vi "NI_cDAQ.vi"(7 "simulazione":bool, 8 "error in (no error)":errorcluster, 10 "banco":i32, 11 "Queue Name":string="NIcDAQ_Q") -> (0 "error out":errorcluster, 2 "Stopped":bool)   [LabVIEW 2019]
uses:
  TypeDef/Cluster NI.ctl
  cDAQ_PLC Folder/controls/StatoAO_cdaq.ctl
  cDAQ_PLC Folder/controls/statoDO_Cdaq.ctl
  cDAQ_PLC Folder/IN_Cluster.ctl
  cDAQ_PLC Folder/OUT_CLUSTER.ctl
  <vilib>/addons/_NISVFA/_Shared subVIs/Controls/svc_Channel Info.ctl
  <vilib>/addons/_NISVFA/_Shared subVIs/Controls/svc_Engineering Units Text Ring.ctl
  <vilib>/addons/_NISVFA/_Shared subVIs/Controls/svc_Weighting Filter Text Ring.ctl
  <vilib>/addons/_NISVFA/_Shared subVIs/Controls/svc_Window.ctl
  TypeDef/DEVICE NAME.ctl
  TypeDef/CLUSTER AI SIM.ctl
  <vilib>/DAQmx/read.llb/DAQmx Read (Counter DBL 1Chan 1Samp).vi
  <vilib>/DAQmx/read.llb/DAQmx Read (Analog 1D Wfm NChan NSamp).vi
  <vilib>/Analysis/baseanly.llb/Mean (DBL).vi
  <vilib>/DAQmx/write.llb/DAQmx Write (Digital 1D Bool NChan 1Samp 1Line).vi
  <vilib>/DAQmx/write.llb/DAQmx Write (Analog 1D DBL NChan 1Samp).vi
  <vilib>/Utility/file.llb/Read From Spreadsheet File (string).vi
  <vilib>/Utility/file.llb/Write To Spreadsheet File (string).vi
  <vilib>/DAQmx/miscellaneous.llb/DAQmx Fill In Error Info.vi
  Globals.vi
  <vilib>/Utility/file.llb/Read From Spreadsheet File (DBL).vi
  <vilib>/Analysis/NI_AALBase.lvlib
  cDAQ_PLC Folder/SubVI/EXIT.vi
  Global allarme combinazione DO.vi
  <vilib>/addons/Sound and Vibration/svt_Calibration/SoundVib_Calibration.lvlib
  <vilib>/measure/NI_MAPro.lvlib
  <vilib>/measure/NI_MABase.lvlib
  rpm nominali global.vi
  <resource>/objmgr/daqmx.rc
  <vilib>/DAQmx/read.llb/DAQmx Read (Analog 1D DBL NChan 1Samp).vi
  <vilib>/DAQmx/read.llb/DAQmx Read (Analog Wfm 1Chan NSamp).vi
  <vilib>/DAQmx/configure/timing.llb/DAQmx Timing (Sample Clock).vi
  <vilib>/addons/Sound and Vibration/svt_Calibration/SVL Scale Voltage to EU (1 Ch).vi
  <vilib>/addons/_NISVFA/_Spectrum Processing/SVFA Spectrum Peak Search (1 Ch).vi
  <vilib>/addons/_NISVFA/_Subset FFT/SVFA Power Spectrum Subset (1 Ch).vi
panel:
  in  "element":dbl[](array[numeric])
  in  "SET AO":bool
  out "EXIT 2":bool=TRUE
  out "error AO 2":errorcluster
  out "# pending insert 4":i32
  out "t ciclo effettivo AO 2":u32
  out "AO cdaq [0-10V]":T1
  out "x-y 2":u32
  out "Array":dbl[](array[numeric])
  out "error DO 2":errorcluster
  out "statoDO 2":T2
  out "# pending insert 3":i32
  out "Numeric 2":i32
  out "stop":bool
  in  "dB On (T)":bool=TRUE
  out "Letture":T3 {"Stato uscite"."AO" format="%f%0.2f"; "AI2" format="%#_6f"; "TC" format="%#_4f"; "AI1" format="%#_6f"}
  out "AO cdaq 4-20mA":T1
  out "Temperature [°C]":T5
  out "Contatori [rpm]":cluster{"RPM 1":dbl, "RPM 2":dbl}
  out "error AO":errorcluster
  out "x-y":u32
  out "# pending insert 2":i32
  out "t ciclo effettivo AO":u32
  out "SampleRate":dbl
  out "subarray":string[](array[string])
  out "all rows":string[][](array[string])
  out "N°samples":i32
  out "appended path":path
  out "SampleMode":i32
  in  "Tab Control":T6(tab)
  in  "ESEGUI SOLO IL VI":bool
  out "LOOP TIME (ms)":u32
  out "Cluster READ":T7 {"AI (4-20mA)"."AI 15" format="%#_6f"; "AI (4-20mA)"."AI 14" format="%#_6f"; "AI (4-20mA)"."AI 13" format="%#_6f"; "AI (4-20mA)"."AI 11" format="%#_6f"; "AI (4-20mA)"."AI 10" format="%#_6f"; "AI (4-20mA)"."AI 9" format="%#_6f"; "AI (4-20mA)"."AI 4" format="%#_6f"; "AI (4-20mA)"."AI 12" format="%#_6f"; "AI (4-20mA)"."AI 0" format="%#_6f"; "AI (4-20mA)"."AI 1" format="%#_6f"; "AI (4-20mA)"."AI 2" format="%#_6f"; "AI (4-20mA)"."AI 3" format="%#_6f"; "AI (4-20mA)"."AI 5" format="%#_6f"; "AI (4-20mA)"."AI 6" format="%#_6f"; "AI (4-20mA)"."AI 7" format="%#_6f"; "AI (4-20mA)"."AI 8" format="%#_6f"; "AI (0-10V)"."AI 31" format="%#_6f"; "AI (0-10V)"."AI 30" format="%#_6f"; "AI (0-10V)"."AI 29" format="%#_6f"; "AI (0-10V)"."AI 28" format="%#_6f"; "AI (0-10V)"."AI 27" format="%#_6f"; "AI (0-10V)"."AI 26" format="%#_6f"; "AI (0-10V)"."AI 25" format="%#_6f"; "AI (0-10V)"."AI 24" format="%#_6f"; "AI (0-10V)"."AI 23" format="%#_6f"; "AI (0-10V)"."AI 22" format="%#_6f"; "AI (0-10V)"."AI 21" format="%#_6f"; "AI (0-10V)"."AI 20" format="%#_6f"; "AI (0-10V)"."AI 19" format="%#_6f"; "AI (0-10V)"."AI 18" format="%#_6f"; "AI (0-10V)"."AI 17" format="%#_6f"; "AI (0-10V)"."AI 16" format="%#_6f"; "AI (0-10V)"."AI 15" format="%#.3f"; "AI (0-10V)"."AI 14" format="%#.3f"; "AI (0-10V)"."AI 13" format="%#.3f"; "AI (0-10V)"."AI 11" format="%#.3f"; "AI (0-10V)"."AI 10" format="%#.3f"; "AI (0-10V)"."AI 9" format="%#.3f"; "AI (0-10V)"."AI 4" format="%#.3f"; "AI (0-10V)"."AI 12" format="%#.3f"; "AI (0-10V)"."AI 0" format="%#.3f"; "AI (0-10V)"."AI 1" format="%#.3f"; "AI (0-10V)"."AI 2" format="%#.3f"; "AI (0-10V)"."AI 3" format="%#.3f"; "AI (0-10V)"."AI 5" format="%#.3f"; "AI (0-10V)"."AI 6" format="%#.3f"; "AI (0-10V)"."AI 7" format="%#.3f"; "AI (0-10V)"."AI 8" format="%#.3f"}
  out "frequency":dbl
  out "error TC":errorcluster
  out "STATO":string
  out "variant":variant
  out "Array nomi moduli":string[](array[string])
  out "Cluster TASK":T9
  in  "lower limit":dbl=1.0 format="%#_13g"
  in  "upper limit":dbl=10000.0 format="%#_13g"
  in  "campioni media rpm":i32=3
  in  "timeout":dbl=0.5 format="%#_13g"
  out "Frequenza":dbl
  out "error in (no error) 2":errorcluster
  out "error out 3":errorcluster
  out "CTR error 2":errorcluster
  out "NI9203":errorcluster caption="error out"
  out "NI9265":errorcluster
  out "CTR TASK":errorcluster caption="error out"
  out "NI9215":errorcluster caption="ni 9215"
  in  "Boolean":bool
  in  "DI.DigFltr.Enable":bool=TRUE
  in  "DI.DigFltr.MinPulseWidth":dbl=6.4e-06
  out "Numeric":i32
  in  "SALVA IMP FILTRI 0-10V":bool
  out "Not filtered 4-20mA":waveform(dbl)[](graph)
  out "Filtered 4-20mA":waveform(dbl)[](graph)
  in  "Impostazioni filtri digitali su canali 4-20mA":T10(array[cluster])=[{"filter?"=FALSE, "low cutoff freq: fl"=0.12500000000000006, "order"=2}, {"filter?"=FALSE, "low cutoff freq: fl"=0.12500000000000006, "order"=2}, {"filter?"=FALSE, "low cutoff freq: fl"=0.12500000000000006, "order"=2}, {"filter?"=FALSE, "low cutoff freq: fl"=0.12500000000000006, "order"=2}, {"filter?"=FALSE, "low cutoff freq: fl"=0.12500000000000006, "order"=2}, {"filter?"=FALSE, "low cutoff freq: fl"=0.12500000000000006, "order"=2}, {"filter?"=FALSE, "low cutoff freq: fl"=0.12500000000000006, "order"=2}, {"filter?"=FALSE, "low cutoff freq: fl"=0.12500000000000006, "order"=2}, {"filter?"=FALSE, "low cutoff freq: fl"=0.12500000000000006, "order"=2}, {"filter?"=FALSE, "low cutoff freq: fl"=0.12500000000000006, "order"=2}, {"filter?"=FALSE, "low cutoff freq: fl"=0.12500000000000006, "order"=2}, {"filter?"=FALSE, "low cutoff freq: fl"=0.12500000000000006, "order"=2}, {"filter?"=FALSE, "low cutoff freq: fl"=0.12500000000000006, "order"=2}, {"filter?"=FALSE, "low cutoff freq: fl"=0.12500000000000006, "order"=2}, {"filter?"=FALSE, "low cutoff freq: fl"=0.12500000000000006, "order"=2}, {"filter?"=FALSE, "low cutoff freq: fl"=0.12500000000000006, "order"=2}] {"low cutoff freq: fl" format="%0.4f"}
  in  "SALVA IMP FILTRI 4-20mA":bool
  in  "Impostazioni filtri digitali su canali 0-10V":T10(array[cluster])=[{"filter?"=FALSE, "low cutoff freq: fl"=0.12500000000000006, "order"=2}, {"filter?"=FALSE, "low cutoff freq: fl"=0.12500000000000006, "order"=2}, {"filter?"=FALSE, "low cutoff freq: fl"=0.12500000000000006, "order"=2}, {"filter?"=FALSE, "low cutoff freq: fl"=0.12500000000000006, "order"=2}, {"filter?"=FALSE, "low cutoff freq: fl"=0.12500000000000006, "order"=2}, {"filter?"=FALSE, "low cutoff freq: fl"=0.12500000000000006, "order"=2}, {"filter?"=FALSE, "low cutoff freq: fl"=0.12500000000000006, "order"=2}, {"filter?"=FALSE, "low cutoff freq: fl"=0.12500000000000006, "order"=2}, {"filter?"=FALSE, "low cutoff freq: fl"=0.12500000000000006, "order"=2}, {"filter?"=FALSE, "low cutoff freq: fl"=0.12500000000000006, "order"=2}, {"filter?"=FALSE, "low cutoff freq: fl"=0.12500000000000006, "order"=2}, {"filter?"=FALSE, "low cutoff freq: fl"=0.12500000000000006, "order"=2}, {"filter?"=FALSE, "low cutoff freq: fl"=0.12500000000000006, "order"=2}, {"filter?"=FALSE, "low cutoff freq: fl"=0.12500000000000006, "order"=2}, {"filter?"=FALSE, "low cutoff freq: fl"=0.12500000000000006, "order"=2}, {"filter?"=FALSE, "low cutoff freq: fl"=0.12500000000000006, "order"=2}] {"low cutoff freq: fl" format="%0.4f"}
  out "Filtered 0-10V":waveform(dbl)[](graph)
  out "Not filtered 0-10V":waveform(dbl)[](graph)
  in  "tone amplitudes":dbl[](array[numeric])=[1.0, 1.0, 1.0, 1.0] format="%.2p"
  in  "tone frequencies":dbl[](array[numeric])=[100.0, 200.0, 300.0, 400.0] format="%.2p"
  in  "averaging parameters":T11={"averaging mode"=enum."Peak hold", "weighting mode"=enum."Exponential", "number of averages"=10, "linear mode"=enum."Auto restart"}
  in  "channel info":T12={"sensor sensitivity"=100.0, "engineering units"=3, "dB reference"=2e-05, "custom label"="EU", "weighting filter"=0, "pregain"=0.0} {"pregain" format="%.2f"; "weighting filter" items=["Linear", "A-weighting", "B-weighting", "C-weighting", "ITU-R 468-4", "Dolby", "CCITT", "C-message", "Wb", "Wc", "Wd", "We", "Wf", "Wh", "Wj", "Wk", "Wm", "AES17 20 kHz lowpass", "AES17 40 kHz lowpass", "AES17 20 kHz highpass", "AES17 40 kHz highpass"]; "dB reference" format="%^.1e"; "engineering units" items=["custom..."=0, "V"=1, "A"=21, "C"=30, "pC"=31, "s"=32, "-"=29, "Pa"=2, "N"=20, "g"=3, "m/s^2"=4, "m/s"=5, "m"=6, "mm/s"=12, "mm"=13, "micron/s"=14, "micron"=15, "in/s^2"=7, "in/s"=8, "in"=9, "mil/s"=10, "mil"=11, "rad/s^2"=16, "rad/s"=17, "rad"=18, "deg/s^2"=26, "deg/s"=27, "deg"=28, "RPM"=22, "cycle/s^2"=23, "Hz"=24, "cycle"=25, "strain"=19]; "sensor sensitivity" format="%#_5f"}
  out "peaks found":i32(listbox)=-1
  out "averages completed":dbl
  out "averaging done":bool
  out "number of peaks":i32
  in  "window":T15 items=["None"=0, "Hanning"=1, "Hamming"=2, "Blackman-Harris"=3, "Exact Blackman"=4, "Blackman"=5, "Flat Top"=6, "4 Term B-Harris "=7, "7 Term B-Harris"=8, "Low Sidelobe"=9, "Force"=64, "Exponential"=65, "Blackman Nuttall"=11, "Triangle"=30, "Bartlett-Hanning"=31, "Bohman"=32, "Parzen"=33, "Welch"=34, "Kaiser"=60, "Dolph-Chebyshev"=61, "Gaussian"=62]
  out "Power Spectrum":cluster{"f0":dbl, "df":dbl, "magnitude":dbl[]}(graph)={"f0"=200.0, "df"=0.5, "magnitude"=[]}
  out "frequency range [Hz]":cluster{"start":dbl, "stop":dbl}={"start"=200.0, "stop"=2000.0} {"stop" min=0.0 format="%.2f"; "start" min=0.0 format="%.2f"}
  in  "peak search settings":T16={"single/multiple"=enum."Single Max Peak", "threshold"=inf} {"threshold" format="%.2f"}
  out "F RPM NOM":dbl
  out "Server_RPM_Nom":dbl
  in  "TOLL F-":dbl=4.0
  in  "toll F+":dbl=1.0
  out "RPM":dbl
  out "detected frequency":dbl format="%.2p"
  in  "number of samples":i32=100000
  in  "rate":dbl=40000.0 format="%0.2f"
  out "x = y?":bool
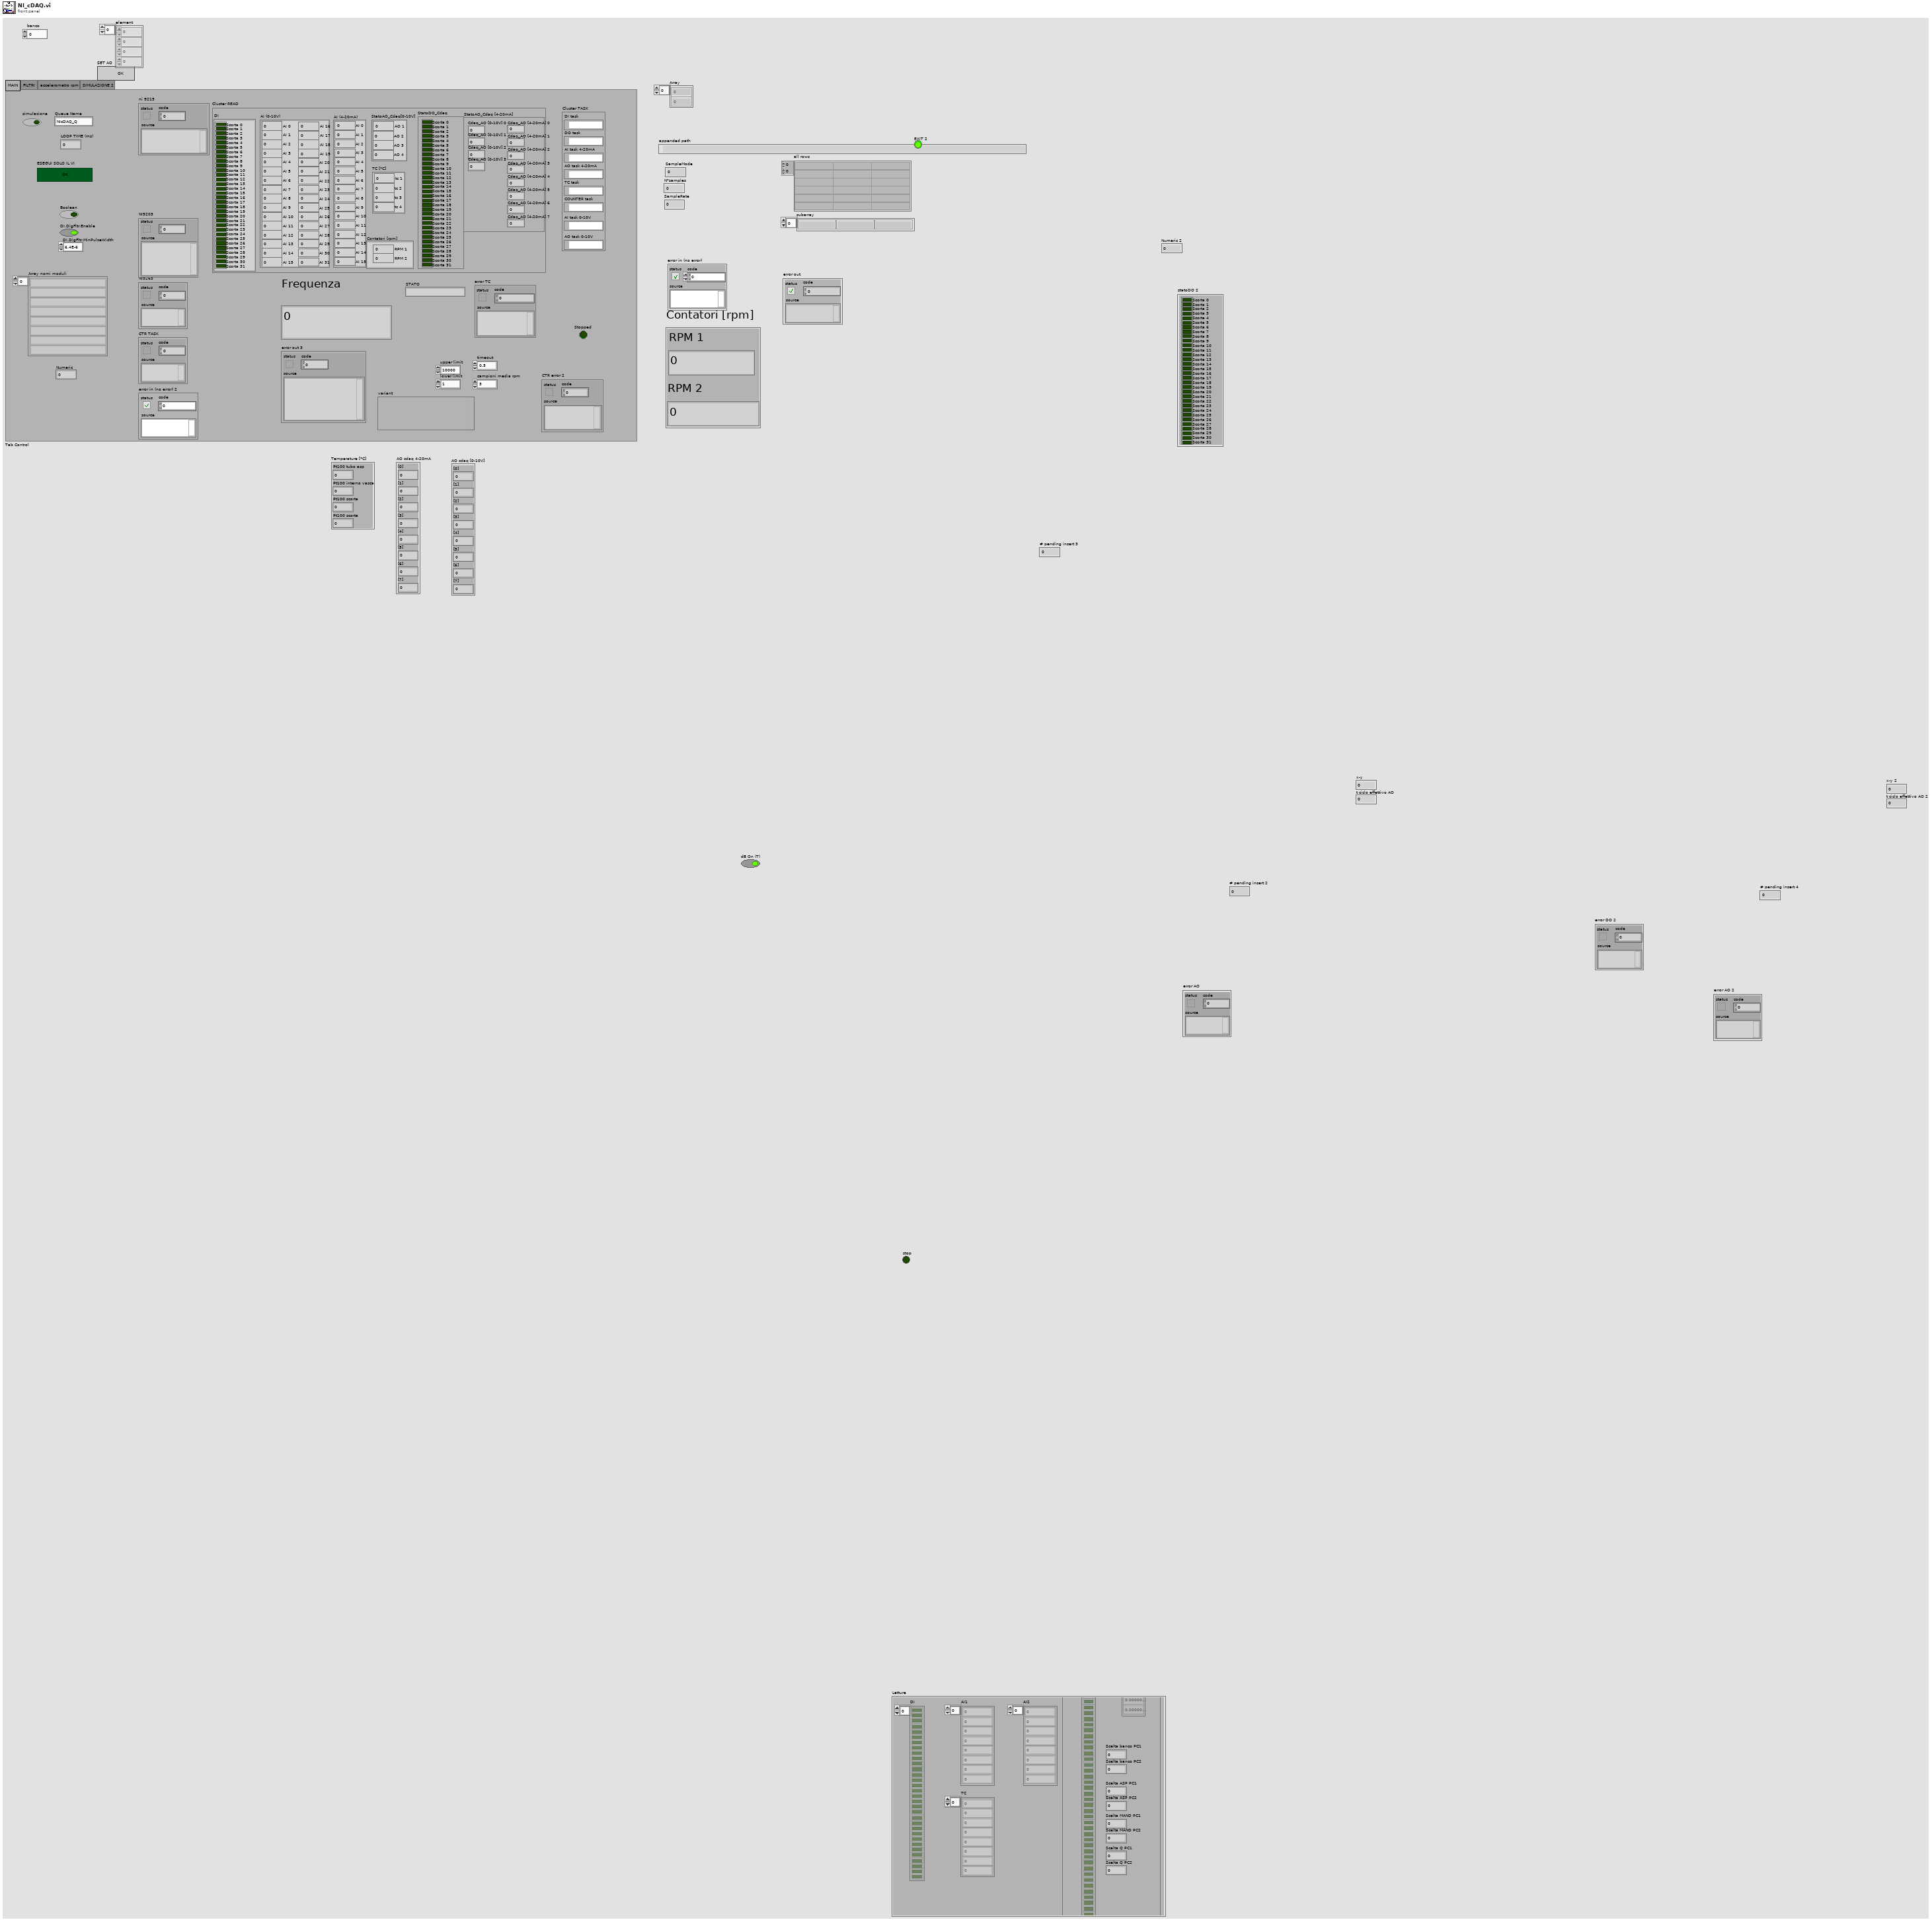
[diagram p1: front panel]
types:
  T1 = cluster{"[0]":dbl, "[1]":dbl, "[2]":dbl, "[3]":dbl, "[4]":dbl, "[5]":dbl, "[6]":dbl, "[7]":dbl}
  T2 = typedef "statoDO_Cdaq.ctl" = cluster{"Scorta 0":bool, "Scorta 1":bool, "Scorta 2":bool, "Scorta 3":bool, "Scorta 4":bool, "Scorta 5":bool, "Scorta 6":bool, "Scorta 7":bool, "Scorta 8":bool, "Scorta 9":bool, "Scorta 10":bool, "Scorta 11":bool, "Scorta 12":bool, "Scorta 13":bool, "Scorta 14":bool, "Scorta 15":bool, "Scorta 16":bool, "Scorta 17":bool, "Scorta 18":bool, "Scorta 19":bool, "Scorta 20":bool, "Scorta 21":bool, "Scorta 22":bool, "Scorta 23":bool, "Scorta 24":bool, "Scorta 25":bool, "Scorta 26":bool, "Scorta 27":bool, "Scorta 28":bool, "Scorta 29":bool, "Scorta 30":bool, "Scorta 31":bool}
  T3 = typedef "IN_Cluster.ctl" = cluster{"DI":bool[], "AI1":dbl[], "TC":dbl[], "AI2":dbl[], "Stato uscite":T4}
  T4 = typedef "OUT_CLUSTER.ctl" = cluster{"DO ":bool[], "AO":dbl[], "Scelta banco PC1":dbl, "Scelta banco PC2":dbl, "Scelta ASP PC1":dbl, "Scelta ASP PC2":dbl, "Scelta MAND PC1":dbl, "Scelta MAND PC2":dbl, "Scelta Q PC1":dbl, "Scelta Q PC2":dbl}
  T5 = cluster{"Pt100 tubo asp":dbl, "Pt100 interno vasca":dbl, "Pt100 scorta":dbl, "Pt100 scorta":dbl}
  T6 = enum32{"MAIN", "FILTRI", "accelerometro rpm", "SIMULAZIONE 2"}
  T7 = typedef "Cluster NI.ctl" = cluster{"AI (0-10V)":cluster{"AI 0":dbl, "AI 1":dbl, "AI 2":dbl, "AI 3":dbl, "AI 4":dbl, "AI 5":dbl, "AI 6":dbl, "AI 7":dbl, "AI 8":dbl, "AI 9":dbl, "AI 10":dbl, "AI 11":dbl, "AI 12":dbl, "AI 13":dbl, "AI 14":dbl, "AI 15":dbl, "AI 16":dbl, "AI 17":dbl, "AI 18":dbl, "AI 19":dbl, "AI 20":dbl, "AI 21":dbl, "AI 22":dbl, "AI 23":dbl, "AI 24":dbl, "AI 25":dbl, "AI 26":dbl, "AI 27":dbl, "AI 28":dbl, "AI 29":dbl, "AI 30":dbl, "AI 31":dbl}, "StatoAO_Cdaq[0-10V]":cluster{"AO 1":dbl, "AO 2":dbl, "AO 3":dbl, "AO 4":dbl}, "Contatori [rpm]":cluster{"RPM 1":dbl, "RPM 2":dbl}, "StatoAO_Cdaq [4-20mA]":T8, "StatoDO_Cdaq":T2, "DI":cluster{"Scorta 0":bool, "Scorta 1":bool, "Scorta 2":bool, "Scorta 3":bool, "Scorta 4":bool, "Scorta 5":bool, "Scorta 6":bool, "Scorta 7":bool, "Scorta 8":bool, "Scorta 9":bool, "Scorta 10":bool, "Scorta 11":bool, "Scorta 12":bool, "Scorta 13":bool, "Scorta 14":bool, "Scorta 15":bool, "Scorta 16":bool, "Scorta 17":bool, "Scorta 18":bool, "Scorta 19":bool, "Scorta 20":bool, "Scorta 21":bool, "Scorta 22":bool, "Scorta 23":bool, "Scorta 24":bool, "Scorta 25":bool, "Scorta 26":bool, "Scorta 27":bool, "Scorta 28":bool, "Scorta 29":bool, "Scorta 30":bool, "Scorta 31":bool}, "AI (4-20mA)":cluster{"AI 0":dbl, "AI 1":dbl, "AI 2":dbl, "AI 3":dbl, "AI 4":dbl, "AI 5":dbl, "AI 6":dbl, "AI 7":dbl, "AI 8":dbl, "AI 9":dbl, "AI 10":dbl, "AI 11":dbl, "AI 12":dbl, "AI 13":dbl, "AI 14":dbl, "AI 15":dbl}, "TC [°C]":cluster{"tc 1":dbl, "tc 2":dbl, "tc 3":dbl, "tc 4":dbl}}
  T8 = typedef "StatoAO_cdaq.ctl" = cluster{"Cdaq_AO [0-10V] 0":dbl, "Cdaq_AO [0-10V] 1":dbl, "Cdaq_AO [0-10V] 2":dbl, "Cdaq_AO [0-10V] 3":dbl, "Cdaq_AO [4-20mA] 0":dbl, "Cdaq_AO [4-20mA] 1":dbl, "Cdaq_AO [4-20mA] 2":dbl, "Cdaq_AO [4-20mA] 3":dbl, "Cdaq_AO [4-20mA] 4":dbl, "Cdaq_AO [4-20mA] 5":dbl, "Cdaq_AO [4-20mA] 6":dbl, "Cdaq_AO [4-20mA] 7":dbl}
  T9 = cluster{"DI task":refnum<k21>, "DO task":refnum<k21>, "AI task 4-20mA":refnum<k21>, "AO task 4-20mA":refnum<k21>, "TC task":refnum<k21>, "COUNTER task":refnum<k21>, "AI task 0-10V":refnum<k21>, "AO task 0-10V":refnum<k21>}
  T10 = cluster{"filter?":bool, "low cutoff freq: fl":dbl, "order":i32}[]
  T11 = cluster{"averaging mode":enum16{"No averaging", "Vector averaging", "RMS averaging", "Peak hold"}, "weighting mode":enum16{"Linear", "Exponential"}, "number of averages":u32, "linear mode":enum16{"One shot", "Auto restart"}}
  T12 = typedef "svc_Channel Info.ctl" = cluster{"sensor sensitivity":dbl, "engineering units":T13, "dB reference":dbl, "custom label":string, "weighting filter":T14, "pregain":dbl}
  T13 = typedef "svc_Engineering Units Text Ring.ctl" = u16
  T14 = typedef "svc_Weighting Filter Text Ring.ctl" = u16
  T15 = typedef "svc_Window.ctl" = u32
  T16 = cluster{"single/multiple":enum16{"Multiple Peaks", "Single Max Peak"}, "threshold":dbl}
  T17 = cluster{"filter?":bool, "low cutoff freq: fl":dbl, "order":i32}
  T18 = typedef "DEVICE NAME.ctl" = enum16{"WT330", "APLUS", "PLC QP", "PLC RACK", "PLC CARICO", "PS", "NI cDAQ", "RESMETER"}
  T19 = enum32{"Invalid", "Standard", "Closed", "Hidden", "Minimized", "Maximized"}
  T20 = enum16{"No averaging", "Vector averaging", "RMS averaging", "Peak hold"}
  T21 = cluster{"Array of elements":cluster{"String":string, "variant":variant}[], "Single element":cluster{"String":string, "variant":variant}, "enque at\nopposite end (F)":bool, "no replications (F)":bool}
  T22 = typedef "CLUSTER AI SIM.ctl" = cluster{"Portata 1":cluster{"Amplitude [mA]":dbl, "Precision %":dbl}, "Portata 2":cluster{"Amplitude [mA]":dbl, "Precision %":dbl}, "Portata 3":cluster{"Amplitude [mA]":dbl, "Precision %":dbl}, "Portata 4":cluster{"Amplitude [mA]":dbl, "Precision %":dbl}, "Pressione 1":cluster{"Amplitude [mA]":dbl, "Precision %":dbl}, "Pressione 2":cluster{"Amplitude [mA]":dbl, "Precision %":dbl}, "Pressione 3":cluster{"Amplitude [mA]":dbl, "Precision %":dbl}, "Pressione 4":cluster{"Amplitude [mA]":dbl, "Precision %":dbl}, "Velocità":cluster{"Amplitude [mA]":dbl, "Precision %":dbl}, "Coppia":cluster{"Amplitude [mA]":dbl, "Precision %":dbl}, "Temperatura 1":cluster{"Amplitude [mA]":dbl, "Precision %":dbl}, "Temperatura 2":cluster{"Amplitude [mA]":dbl, "Precision %":dbl}, "Livello":cluster{"Amplitude [mA]":dbl, "Precision %":dbl}, "Pressione serbatoio":cluster{"Amplitude [mA]":dbl, "Precision %":dbl}}
  T23 = cluster{"DI task":refnum<k21>, "DO task":refnum<k21>, "AI task 4-20mA":refnum<k21>, "AO task":refnum<k21>, "TC task":refnum<k21>, "COUNTER task":refnum<k21>, "AI task 0-10V":refnum<k21>}
  T24 = typedef "svc_Spectrum Info.ctl" = cluster{"channel name":string, "description":string, "x-axis units":T25, "spectral info":cluster{"spectrum type":T26, "linear/dB":enum16{"linear", "dB"}, "window":u16, "window size":i32, "FFT size":i32}, "engineering units":T13, "custom label":string, "dB reference [EU]":dbl, "peak units":enum16{"rms", "peak", "peak-peak"}, "weighting filter":T14, "spectral density?":bool, "unit label":string, "spectrum skewed?":bool, "complimentary spectrum units":T27}
  T25 = typedef "svc_X-Axis Units.ctl" = u16
  T26 = typedef "svc_Spectrum Type.ctl" = enum16{"FFT Spectrum [complex]", "Amplitude [Magnitude]", "Power [Magnitude^2]", "Cross Spectrum [complex]", "Frequency Response [Complex]"}
  T27 = typedef "svc_Complimentary Spectrum Units.ctl" = enum16{"none", "radians", "degrees", "cycles", "imaginary"}
  T28 = cluster{"data[0]":dbl, "data[1]":dbl, "data[2]":dbl, "data[3]":dbl}
  T29 = cluster{"Array[0]":dbl, "Array[1]":dbl, "Array[2]":dbl, "Array[3]":dbl, "Array[4]":dbl, "Array[5]":dbl, "Array[6]":dbl, "Array[7]":dbl, "Array[8]":dbl, "Array[9]":dbl, "Array[10]":dbl, "Array[11]":dbl, "Array[12]":dbl, "Array[13]":dbl, "Array[14]":dbl, "Array[15]":dbl}
  T30 = cluster{"[0]":dbl, "[1]":dbl, "[2]":dbl, "[3]":dbl, "[4]":dbl, "[5]":dbl, "[6]":dbl, "[7]":dbl, "[8]":dbl, "[9]":dbl, "[10]":dbl, "[11]":dbl, "[12]":dbl, "[13]":dbl, "[14]":dbl, "[15]":dbl, "[16]":dbl, "[17]":dbl, "[18]":dbl, "[19]":dbl, "[20]":dbl, "[21]":dbl, "[22]":dbl, "[23]":dbl, "[24]":dbl, "[25]":dbl, "[26]":dbl, "[27]":dbl, "[28]":dbl, "[29]":dbl, "[30]":dbl, "[31]":dbl}
  T31 = cluster{"Amplitude [mA]":dbl, "Precision %":dbl}[]
  T32 = cluster{"[0]":bool, "[1]":bool, "[2]":bool, "[3]":bool, "[4]":bool, "[5]":bool, "[6]":bool, "[7]":bool, "[8]":bool, "[9]":bool, "[10]":bool, "[11]":bool, "[12]":bool, "[13]":bool, "[14]":bool, "[15]":bool, "[16]":bool, "[17]":bool, "[18]":bool, "[19]":bool, "[20]":bool, "[21]":bool, "[22]":bool, "[23]":bool, "[24]":bool, "[25]":bool, "[26]":bool, "[27]":bool, "[28]":bool, "[29]":bool, "[30]":bool, "[31]":bool}
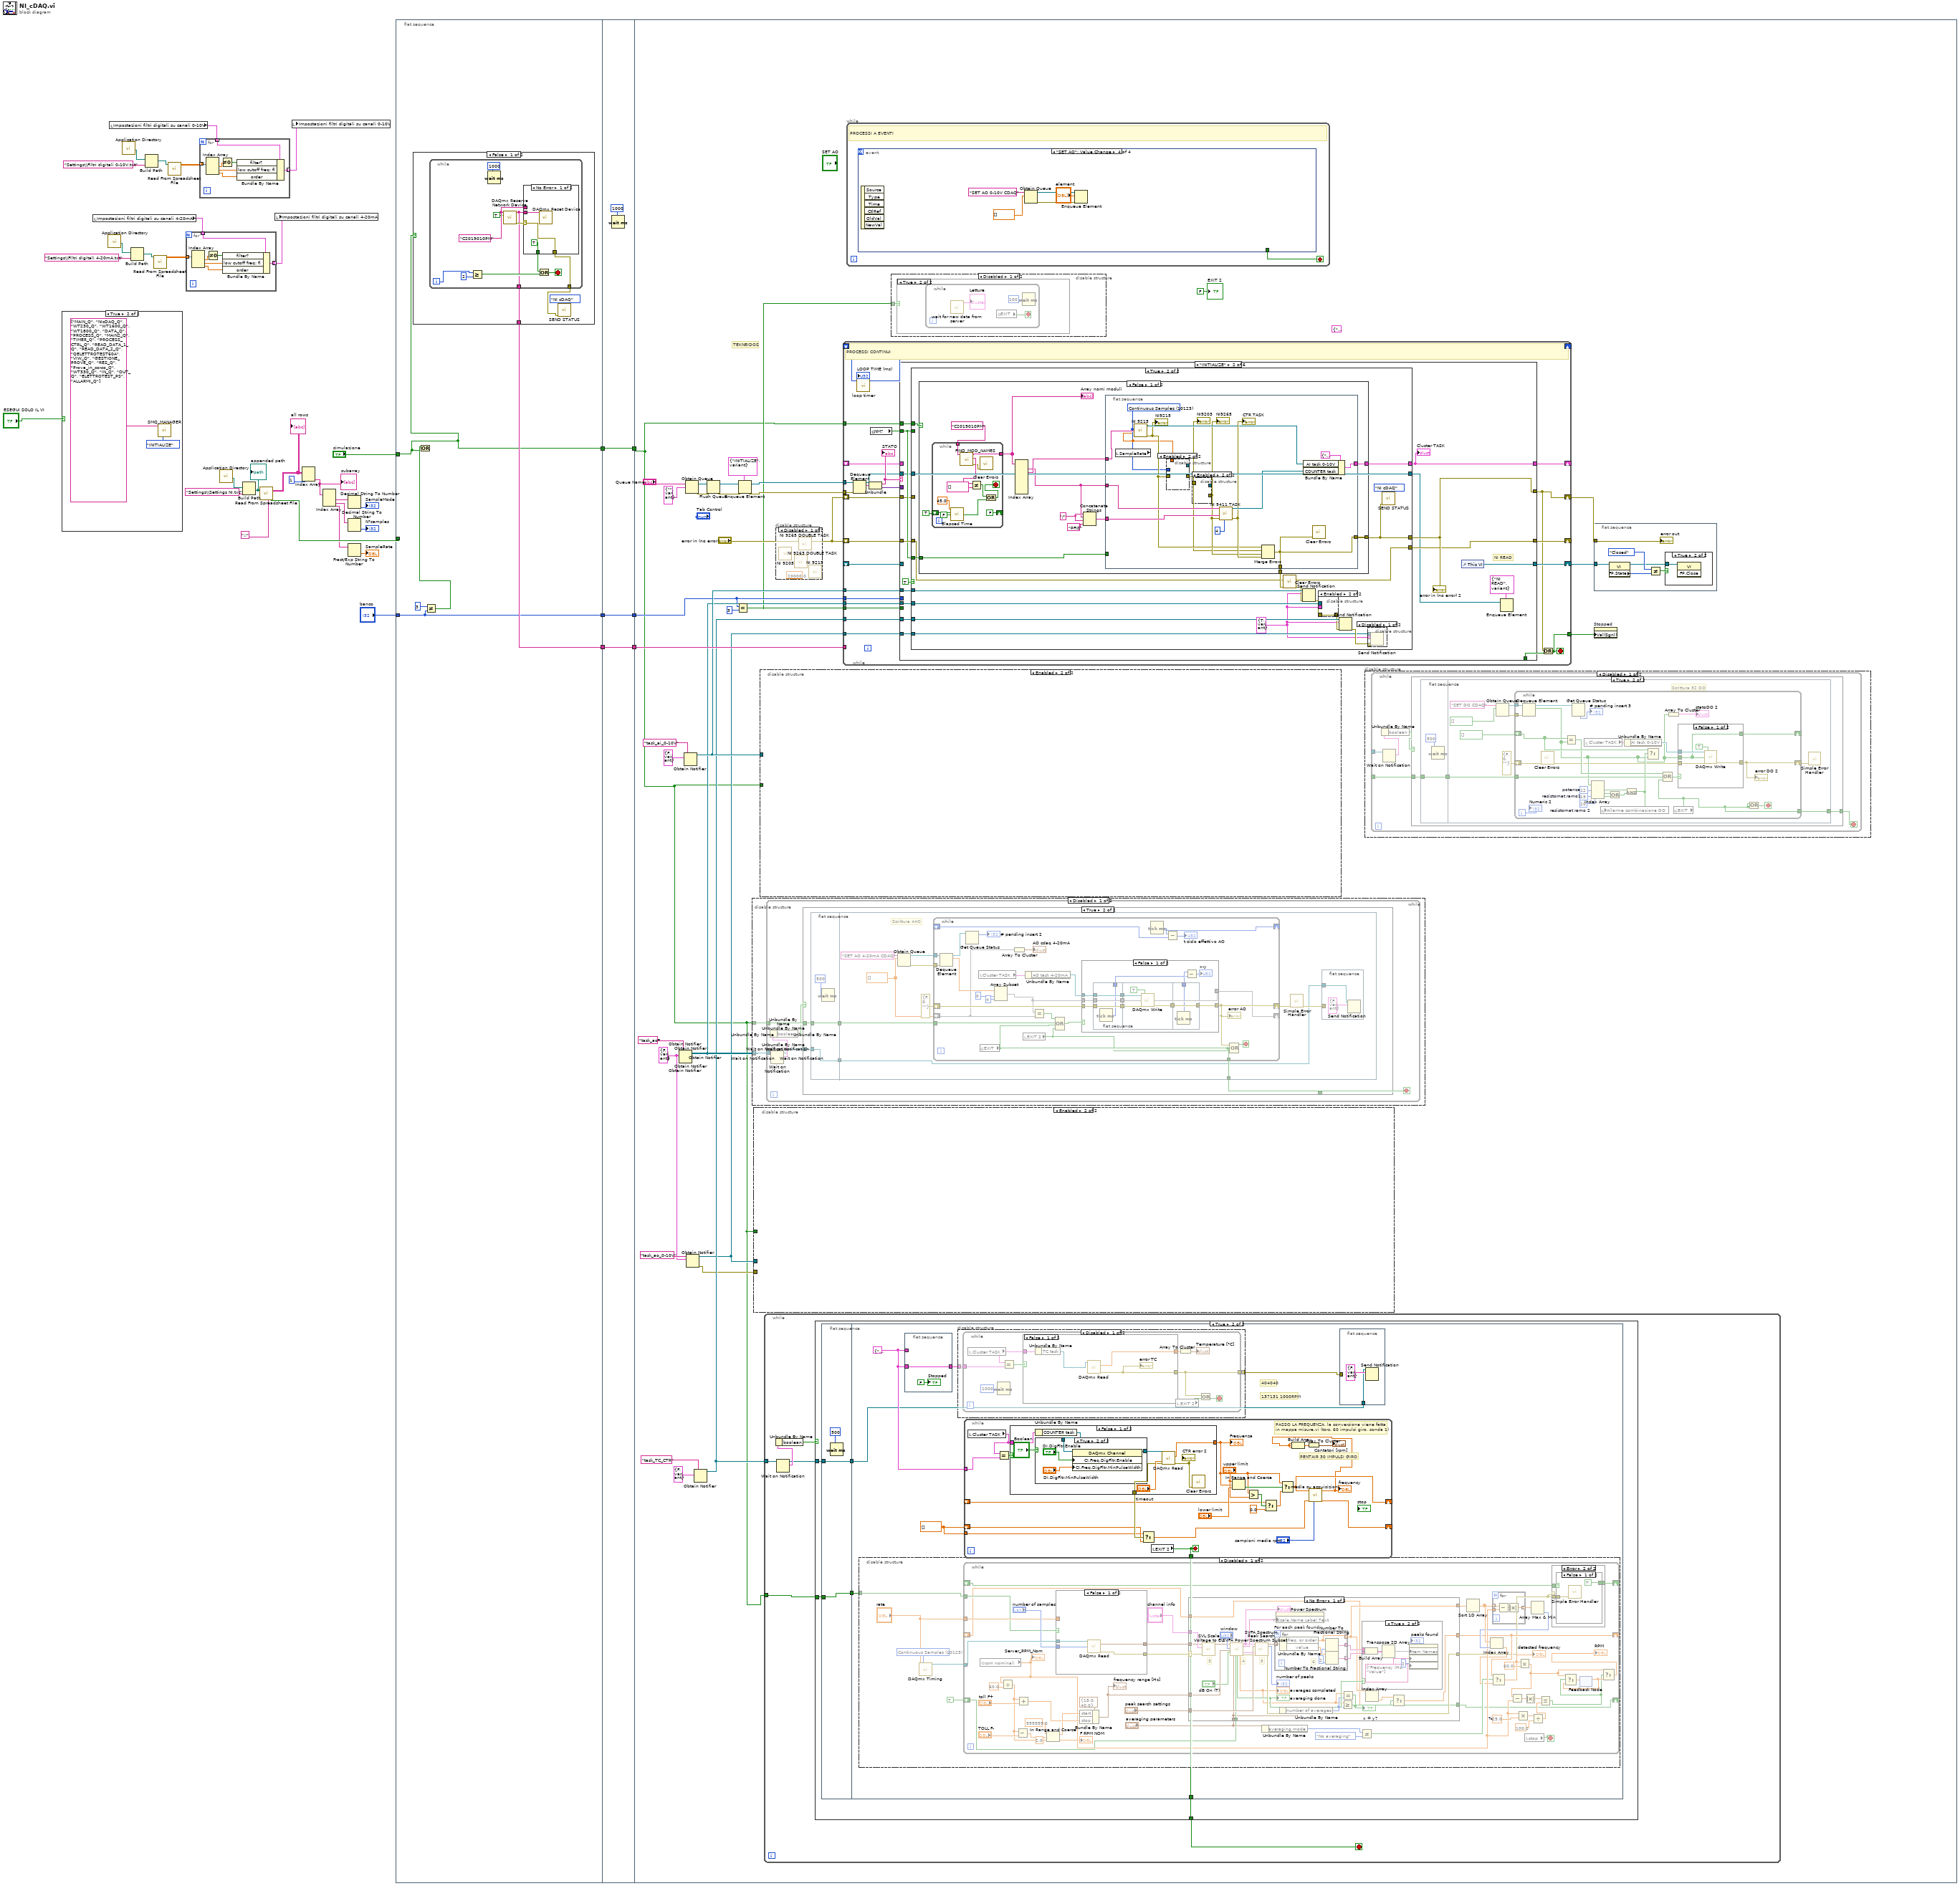
[diagram p0: block diagram]
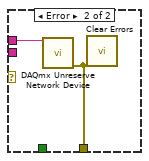
[diagram p3: hidden frame]
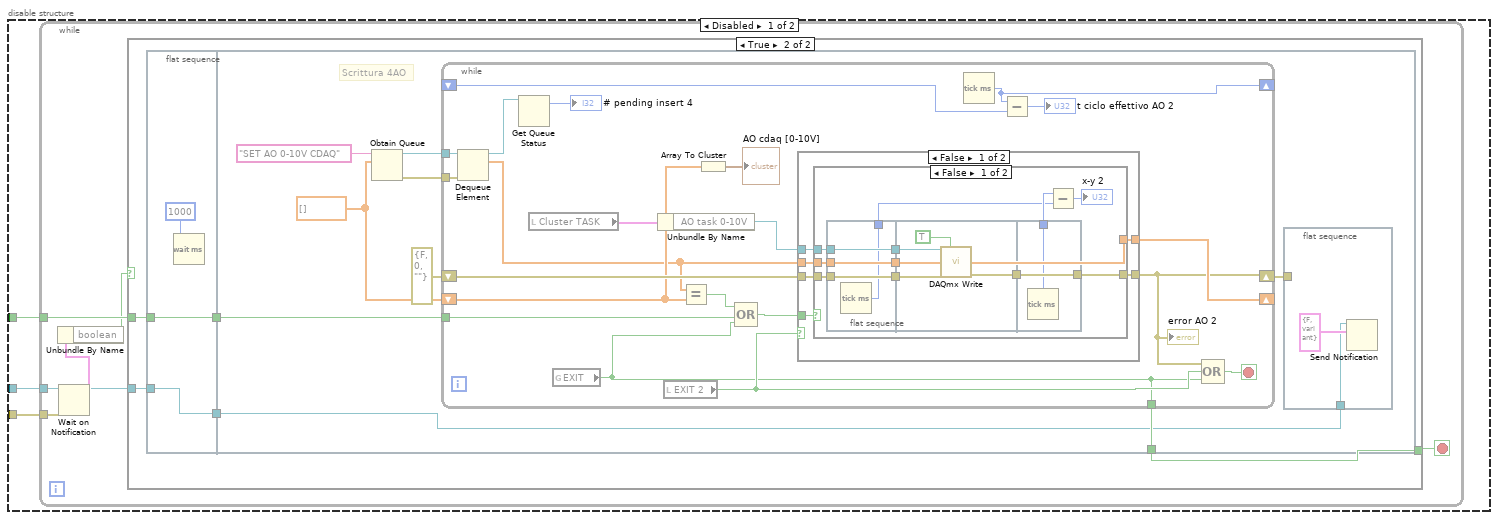
[diagram p5: hidden frame]
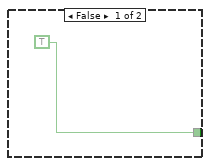
[diagram p6: hidden frame]
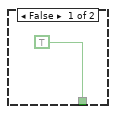
[diagram p9: hidden frame]
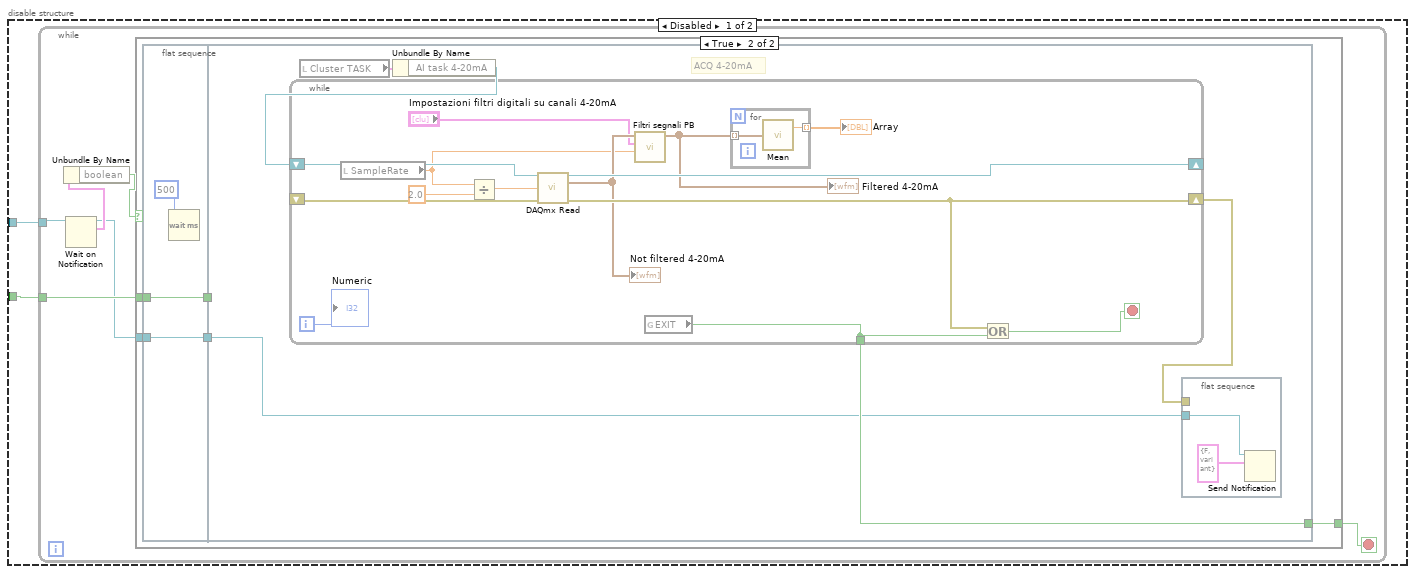
[diagram p12: hidden frame]
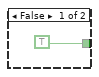
[diagram p13: hidden frame]
diagram:
  n1 = case shown="True" "ESEGUI SOLO IL VI" {
    frame False {
    }
    frame True {
      n2 = call "SMQ_MANAGER.vi"("Function"=enum16{"INITIALIZE", "ENQUEUE", "STOP ALL"}."INITIALIZE", "Queue array"=string[] ["MAIN_Q", "NIcDAQ_Q", "WT230_Q", "WT1600_Q", "WT1800_Q", "DATA_Q", "PROCESS_Q", "MAIN2_Q", "TIMER_Q", "PROCESS_CTRL_Q", "READ_DATA_1_Q", "READ_DATA_2_Q", "QELETTROTEST60A", "VIW_Q", "GESTIONE_PROVE_Q", "RES_Q", "Prova_in_corso_Q", "WT330_Q", "IN_Q", "OUT_Q", "ELETTROTEST_PS", "ALLARMI_Q"]) -> ()  [unwired: 9 in, 1 out]
    }
  }
  n3 = local read "Impostazioni filtri digitali su canali 4-20mA"() -> (w18:T10)
  n4 = call <vilib>:"Application Directory.vi"() -> ("Application Directory"=w22:path)
  n5 = local read "Impostazioni filtri digitali su canali 0-10V"() -> (w7:T10)
  n6 = call <vilib>:"Application Directory.vi"() -> ("Application Directory"=w3:path)
  n7 = Build Path(base path=w22, name or relative path="Settings\\Filtri digitali 4-20mA.txt") -> (appended path=w20:path)
  n8 = Build Path(base path=w3, name or relative path="Settings\\Filtri digitali 0-10V.txt") -> (appended path=w5:path)
  n9 = call-poly <vilib>:"Read From Spreadsheet File.vi"("file path (dialog if empty)"=w20) -> ("all rows"=w19:dbl[][])  [unwired: 6 in, 4 out]
  n10 = call-poly <vilib>:"Read From Spreadsheet File.vi"("file path (dialog if empty)"=w5) -> ("all rows"=w6:dbl[][])  [unwired: 6 in, 4 out]
  n11 = for {
    tunnel: w19 -> [w44] mode=indexing
    tunnel: w18 -> [w43] mode=indexing
    tunnel: [w38] -> w17 mode=indexing
    n12 = Index Array(array=w44) -> (element #1=w42:dbl, element #2=w40:dbl, element #3=w39:dbl)  [unwired: 3 in]
    n13 = Not Equal To 0?(x=w42) -> (x != 0?=w41:bool)
    n14 = Bundle By Name(cluster=w43, "filter?"=w41, "low cutoff freq: fl"=w40, "order"=w39) -> (w38:T17)
  }
  n15 = for {
    tunnel: w6 -> [w51] mode=indexing
    tunnel: w7 -> [w50] mode=indexing
    tunnel: [w45] -> w8 mode=indexing
    n16 = Index Array(array=w51) -> (element #1=w49:dbl, element #2=w47:dbl, element #3=w46:dbl)  [unwired: 3 in]
    n17 = Not Equal To 0?(x=w49) -> (x != 0?=w48:bool)
    n18 = Bundle By Name(cluster=w50, "filter?"=w48, "low cutoff freq: fl"=w47, "order"=w46) -> (w45:T17)
  }
  n19 = call <vilib>:"Application Directory.vi"() -> ("Application Directory"=w30:path)
  n20 = Build Path(base path=w30, name or relative path="Settings\\Settings NI.txt") -> (appended path=w32:path)
  "appended path" <- w32
  n21 = call-poly <vilib>:"Read From Spreadsheet File.vi"("delimiter (\\t)"="::" ("delimiter (\\t)"), "file path (dialog if empty)"=w32) -> ("EOF?"=w29:bool, "all rows"=w28:string[][])  [unwired: 5 in, 3 out]
  "all rows" <- w28
  n22 = local write "Impostazioni filtri digitali su canali 4-20mA"(w17) -> ()
  n23 = local write "Impostazioni filtri digitali su canali 0-10V"(w8) -> ()
  n24 = Index Array(array=w28, index (col)=1 ("disabled index (col)")) -> (element=w26:string[])  [unwired: 1 in]
  "subarray" <- w26
  n25 = Index Array(array=w26) -> (element #1=w25:string, element #2=w24:string, element #3=w23:string)  [unwired: 3 in]
  n26 = Decimal String To Number(string=w25) -> (number=→"SampleMode":i32)  [unwired: 2 in, 1 out]
  n27 = Decimal String To Number(string=w24) -> (number=→"N°samples":i32)  [unwired: 2 in, 1 out]
  n28 = Fract/Exp String To Number(string=w23) -> (number=→"SampleRate":dbl)  [unwired: 3 in, 1 out]
  n29 = flat-sequence {
    tunnel: [w52] -> w15
    tunnel: "simulazione" -> [w52]
    tunnel: w29 -> [_]
    tunnel: [w56] -> w13
    tunnel: "banco" -> [w55]
    tunnel: [w55] -> w11
    tunnel: w15 -> [w79]
    tunnel: [w79] -> w14
    tunnel: w13 -> [w78]
    tunnel: [w78] -> w12
    tunnel: w11 -> [w77]
    tunnel: [w77] -> w10
    tunnel: w14 -> [w82]
    tunnel: w12 -> [w110]
    tunnel: w10 -> [w102]
    frame #0 {
      n30 = case shown="False" w52 {
        tunnel: [w59 _] -> w56
        frame False {
          n31 = while {
            tunnel: [w63] -> w59
            tunnel: [w60] -> w57
            i -> [w68]
            stop <- w65 stop-if-true
            w62 = "C2019010PM" ("RICERCA cDAQ")
            n32 = Greater Or Equal?(x=w68, y=2) -> (x >= y?=w66:bool)
            n33 = Wait (ms)(milliseconds to wait=u32 1000) -> ()  [unwired: 1 out]
            n34 = call <vilib>:"DAQmx Reserve Network Device.vi"("device in"=w62, "override reservation?"=TRUE) -> ("device out"=w63:tag, "error out"=w70:errorcluster)  [unwired: 12 in]
            n35 = case shown="No Error" w70 {
              selector: w70 -> [w71 _]
              tunnel: w62 -> [_ w75]
              tunnel: [TRUE _] -> w69
              tunnel: w63 -> [w72 _]
              tunnel: [w71 w74] -> w60
              frame No Error {
                n36 = call <vilib>:"DAQmx Reset Device.vi"("device in"=w72) -> ()  [unwired: 14 in, 1 out]
              }
              frame Error {
                n37 = call <vilib>:"DAQmx Unreserve Network Device.vi"("device in"=w75) -> ("error out"=w74:errorcluster)  [unwired: 13 in, 1 out]
                n38 = call <vilib>:"Clear Errors.vi"("error in (no error)"=w74) -> ()  [unwired: 5 in, 2 out]
              }
            }
            n39 = Or(x=w69, y=w66) -> (x .or. y?=w65:bool)
          }
          n40 = call "SEND STATUS.vi"("ELEMENT"=DEVICE_NAME."NI cDAQ", "error in (no error)"=w57) -> ()  [unwired: 9 in, 1 out]
        }
        frame True {
        }
      }
      n41 = Not Equal?(x=3, y=w55) -> (x != y?=w53:bool)
      n42 = Or(x=w53, y=w52) -> ()  [unwired: 1 out]
    }
    frame #1 {
      n43 = Wait (ms)(milliseconds to wait=u32 1000) -> ()  [unwired: 1 out]
    }
    frame #2 {
      (unwired) T23 {"DI task"="", "DO task"="", "AI task 4-20mA"="", "AO task"="", "TC task"="", "COUNTER task"="", "AI task 0-10V"=""}
      w84 = cluster{"boolean":bool, "variant":variant} {"boolean"=FALSE, "variant"=variant} ("notification")
      # "TEKNEIDOS"
      n44 = Obtain Notifier(name (unnamed)="task_ao" ("Notifier Name"), notification data type=w84) -> (notifier out=w91:refnum<notifier>)  [unwired: 2 in, 2 out]
      n45 = Obtain Notifier(name (unnamed)="task_ao" ("Notifier Name"), notification data type=cluster{"boolean":bool, "variant":variant} {"boolean"=FALSE, "variant"=variant} ("notification")) -> (notifier out=w92:refnum<notifier>)  [unwired: 2 in, 2 out]
      n46 = Obtain Notifier(name (unnamed)="task_ao" ("Notifier Name"), notification data type=cluster{"boolean":bool, "variant":variant} {"boolean"=FALSE, "variant"=variant} ("notification")) -> (notifier out=w97:refnum<notifier>)  [unwired: 2 in, 2 out]
      n47 = Obtain Notifier(name (unnamed)="task_ao" ("Notifier Name"), notification data type=cluster{"boolean":bool, "variant":variant} {"boolean"=FALSE, "variant"=variant} ("notification")) -> (notifier out=w100:refnum<notifier>)  [unwired: 2 in, 2 out]
      n48 = Obtain Notifier(name (unnamed)="task_ao" ("Notifier Name"), notification data type=cluster{"boolean":bool, "variant":variant} {"boolean"=FALSE, "variant"=variant} ("notification")) -> (notifier out=w104:refnum<notifier>)  [unwired: 2 in, 2 out]
      n49 = Obtain Notifier(name (unnamed)="task_ai_0-10V" ("Notifier Name"), notification data type=cluster{"boolean":bool, "variant":variant} {"boolean"=FALSE, "variant"=variant} ("notification")) -> (notifier out=w107:refnum<notifier>)  [unwired: 2 in, 2 out]
      n50 = Obtain Queue(name (unnamed)="Queue Name", element data type=cluster{"String":string, "variant":variant} {"String"="", "variant"=variant} ("element")) -> (queue out=w115:refnum<queue>, error out=w114:errorcluster)  [unwired: 3 in, 1 out]
      n51 = Obtain Notifier(name (unnamed)="task_ao_0-10V", notification data type=w84) -> (notifier out=w83:refnum<notifier>, error out=w85:errorcluster)  [unwired: 2 in, 1 out]
      n52 = Obtain Notifier(name (unnamed)="task_TC_CTR" ("Notifier Name"), notification data type=cluster{"boolean":bool, "variant":variant} {"boolean"=FALSE, "variant"=variant} ("notification")) -> (notifier out=w87:refnum<notifier>)  [unwired: 2 in, 2 out]
      n53 = Flush Queue(queue=w115, error in (no error)=w114) -> (queue out=w113:refnum<queue>, error out=w112:errorcluster)  [unwired: 1 out]
      n54 = Equal?(x=w102, y=3) -> (x = y?=w101:bool)
      n55 = Enqueue Element(queue=w113, element=cluster{"String":string, "variant":variant} {"String"="INITIALIZE", "variant"=variant}, error in (no error)=w112) -> (queue out=w118:refnum<queue>, error out=w117:errorcluster)  [unwired: 1 in, 1 out]
      n56 = disable-structure shown="Disabled" {
        disable-tunnel: w104 -> [w211 _]
        disable-tunnel: w100 -> [w210 _]
        disable-tunnel: w97 -> [w209 _]
        disable-tunnel: w92 -> [w208 _]
        disable-tunnel: w91 -> [w207 _]
        disable-tunnel: w82 -> [w206 _]
        frame Disabled {
          n57 = while {
            tunnel: w206 -> [w225]
            tunnel: w211 -> [w221]
            tunnel: w210 -> [w220]
            tunnel: w209 -> [w218]
            tunnel: w208 -> [w215]
            tunnel: w207 -> [w214]
            stop <- w224 stop-if-true
            n58 = Wait on Notification(notifier=w214) -> (notifier out=w212:refnum<notifier>, notification=w213:cluster{"boolean":bool, "variant":variant})  [unwired: 3 in, 2 out]
            n59 = Unbundle By Name(w213) -> ()  [unwired: 1 out]
            n60 = Wait on Notification(notifier=w215) -> (notification=w216:cluster{"boolean":bool, "variant":variant})  [unwired: 3 in, 3 out]
            n61 = Unbundle By Name(w216) -> ()  [unwired: 1 out]
            n62 = Wait on Notification(notifier=w218) -> (notification=w217:cluster{"boolean":bool, "variant":variant})  [unwired: 3 in, 3 out]
            n63 = Unbundle By Name(w217) -> ()  [unwired: 1 out]
            n64 = Wait on Notification(notifier=w220) -> (notification=w219:cluster{"boolean":bool, "variant":variant})  [unwired: 3 in, 3 out]
            n65 = Unbundle By Name(w219) -> ()  [unwired: 1 out]
            n66 = Wait on Notification(notifier=w221) -> (notification=w223:cluster{"boolean":bool, "variant":variant})  [unwired: 3 in, 3 out]
            n67 = Unbundle By Name(w223) -> ("boolean"=w222:bool)
            n68 = case shown="True" w222 {
              tunnel: w225 -> [_ w230]
              tunnel: [TRUE w229] -> w224
              tunnel: w212 -> [_ w227]
              frame False {
              }
              frame True {
                n69 = flat-sequence {
                  tunnel: w230 -> [w234]
                  tunnel: [w234] -> w231
                  tunnel: [w232] -> w228
                  tunnel: w227 -> [w232]
                  tunnel: w231 -> [w240]
                  tunnel: [w238] -> w229
                  tunnel: w228 -> [w235]
                  frame #0 {
                    n70 = Wait (ms)(milliseconds to wait=u32 500) -> ()  [unwired: 1 out]
                  }
                  frame #1 {
                    w244 = dbl[] []
                    # "Scrittura 4AO"
                    n71 = Obtain Queue(name (unnamed)="SET AO 4-20mA CDAQ", element data type=w244) -> (queue out=w243:refnum<queue>, error out=w242:errorcluster)  [unwired: 3 in, 1 out]
                    n72 = while {
                      shift-right: [w266] -> w239
                      shift-left: errorcluster {"status"=FALSE, "code"=0, "source"=""} ("error out") -> [w270]
                      tunnel: w243 -> [w269]
                      tunnel: w242 -> [w268]
                      tunnel: w240 -> [w264]
                      shift-right: [w263] -> _
                      shift-left: w244 -> [w262]
                      shift-right: [w259] -> _
                      shift-left: _ -> [w260]
                      tunnel: [w257] -> w238
                      stop <- w258 stop-if-true
                      n73 = Dequeue Element(queue=w269, error in (no error)=w268) -> (queue out=w267:refnum<queue>, element=w251:dbl[])  [unwired: 1 in, 2 out]
                      n74 = Get Queue Status(queue=w267) -> (# elements in queue=→"# pending insert 2":i32)  [unwired: 2 in, 7 out]
                      n75 = local read "Cluster TASK"() -> (w253:T9)
                      n76 = global read "EXIT.vi" "EXIT"() -> (w257:bool)
                      n77 = Array Subset(array=w251, index=0, length=4) -> (w250:dbl[])
                      n78 = Array To Cluster(array=w262) -> (cluster=→"AO cdaq 4-20mA":T1)
                      n79 = local read "EXIT 2"() -> (w247:bool)
                      n80 = Unbundle By Name(w253) -> ("AO task 4-20mA"=w252:refnum<k21>)
                      n81 = Equal?(x=w250, y=w262) -> (x = y?=w254:bool)
                      n82 = Compound Arithmetic op=OR(w254, w264, w257, w247) -> (w255:bool)
                      n83 = case shown="False" w255 {
                        tunnel: w252 -> [w281 _]
                        tunnel: w270 -> [w280 w293]
                        tunnel: [w279 w293] -> w266
                        tunnel: w250 -> [w278 w294]
                        tunnel: [w278 w294] -> w263
                        frame False {
                          n84 = flat-sequence {
                            tunnel: w278 -> [w283]
                            tunnel: w280 -> [w284]
                            tunnel: w281 -> [w285]
                            tunnel: [w285] -> w277
                            tunnel: [w284] -> w276
                            tunnel: [w283] -> w275
                            tunnel: [w282] -> w272
                            tunnel: w277 -> [w290]
                            tunnel: w276 -> [w289]
                            tunnel: w275 -> [w287]
                            tunnel: [w288] -> w274
                            tunnel: [w292] -> w279
                            tunnel: w274 -> [w292]
                            tunnel: [w291] -> w273
                            frame #0 {
                              n85 = Tick Count (ms)() -> (millisecond timer value=w282:u32)
                            }
                            frame #1 {
                              n86 = call-poly <vilib>:"DAQmx Write.vi"("task/channels in"=w290, "auto start"=TRUE, "data"=w287, "error in"=w289) -> ("error out"=w288:errorcluster)  [unwired: 9 in, 2 out]
                            }
                            frame #2 {
                              n87 = Tick Count (ms)() -> (millisecond timer value=w291:u32)
                            }
                          }
                          n88 = Subtract(x=w273, y=w272) -> (x-y=→"x-y":u32)
                        }
                        frame True {
                        }
                      }
                      "error AO" <- w266
                      n89 = Tick Count (ms)() -> (millisecond timer value=w259:u32)
                      n90 = Subtract(x=w259, y=w260) -> (x-y=→"t ciclo effettivo AO":u32)
                      n91 = Compound Arithmetic op=OR(w266, w257, w247) -> (w258:bool)
                    }
                    n92 = call <vilib>:"Simple Error Handler.vi"("error in (no error)"=w239) -> ("error out"=w236:errorcluster)  [unwired: 4 in, 4 out]
                    n93 = flat-sequence {
                      tunnel: w235 -> [w245]
                      tunnel: w236 -> [_]
                      frame #0 {
                        n94 = Send Notification(notification=cluster{"boolean":bool, "variant":variant} {"boolean"=FALSE, "variant"=variant}, notifier=w245) -> ()  [unwired: 1 in, 2 out]
                      }
                    }
                  }
                }
              }
            }
          }
        }
        frame Enabled {
        }
      }
      n95 = disable-structure shown="Enabled" {
        disable-tunnel: w85 -> [w125 _]
        disable-tunnel: w83 -> [w124 _]
        disable-tunnel: w82 -> [w123 _]
        frame Disabled {
          n96 = while {
            tunnel: w123 -> [w132]
            tunnel: w124 -> [w130]
            tunnel: w125 -> [w127]
            stop <- w131 stop-if-true
            n97 = Wait on Notification(notifier=w130, error in (no error)=w127) -> (notifier out=w126:refnum<notifier>, notification=w129:cluster{"boolean":bool, "variant":variant})  [unwired: 2 in, 2 out]
            n98 = Unbundle By Name(w129) -> ("boolean"=w128:bool)
            n99 = case shown="True" w128 {
              tunnel: w132 -> [_ w137]
              tunnel: [TRUE w136] -> w131
              tunnel: w126 -> [_ w134]
              frame False {
              }
              frame True {
                n100 = flat-sequence {
                  tunnel: w137 -> [w141]
                  tunnel: [w141] -> w138
                  tunnel: [w139] -> w135
                  tunnel: w134 -> [w139]
                  tunnel: w138 -> [w146]
                  tunnel: [w144] -> w136
                  tunnel: w135 -> [w142]
                  frame #0 {
                    n101 = Wait (ms)(milliseconds to wait=u32 1000) -> ()  [unwired: 1 out]
                  }
                  frame #1 {
                    w150 = dbl[] []
                    # "Scrittura 4AO"
                    n102 = Obtain Queue(name (unnamed)="SET AO 0-10V CDAQ", element data type=w150) -> (queue out=w149:refnum<queue>, error out=w148:errorcluster)  [unwired: 3 in, 1 out]
                    n103 = while {
                      shift-right: [w153] -> w145
                      shift-left: errorcluster {"status"=FALSE, "code"=0, "source"=""} ("error out") -> [w173]
                      tunnel: w149 -> [w172]
                      tunnel: w148 -> [w171]
                      tunnel: w146 -> [w169]
                      shift-right: [w166] -> _
                      shift-left: w150 -> [w165]
                      shift-right: [w162] -> _
                      shift-left: _ -> [w163]
                      tunnel: [w157] -> w144
                      stop <- w155 stop-if-true
                      n104 = Dequeue Element(queue=w172, error in (no error)=w171) -> (queue out=w156:refnum<queue>, element=w160:dbl[])  [unwired: 1 in, 2 out]
                      n105 = Get Queue Status(queue=w156) -> (# elements in queue=→"# pending insert 4":i32)  [unwired: 2 in, 7 out]
                      n106 = local read "Cluster TASK"() -> (w154:T9)
                      n107 = global read "EXIT.vi" "EXIT"() -> (w157:bool)
                      n108 = Unbundle By Name(w154) -> ("AO task 0-10V"=w161:refnum<k21>)
                      n109 = local read "EXIT 2"() -> (w158:bool)
                      n110 = Equal?(x=w160, y=w165) -> (x = y?=w167:bool)
                      n111 = Array To Cluster(array=w165) -> (cluster=→"AO cdaq [0-10V]":T1)
                      n112 = Compound Arithmetic op=OR(w167, w169, w157) -> (w168:bool)
                      n113 = case shown="False" w158 {
                        tunnel: w173 -> [w179 w204]
                        tunnel: [w178 w204] -> w153
                        tunnel: w168 -> [w177 _]
                        tunnel: [w176 w205] -> w166
                        tunnel: w161 -> [w175 _]
                        tunnel: w160 -> [w174 w205]
                        frame False {
                          n114 = case shown="False" w177 {
                            tunnel: w175 -> [w190 _]
                            tunnel: w179 -> [w189 w202]
                            tunnel: [w188 w202] -> w178
                            tunnel: w174 -> [w187 w203]
                            tunnel: [w187 w203] -> w176
                            frame False {
                              n115 = flat-sequence {
                                tunnel: w187 -> [w192]
                                tunnel: w189 -> [w193]
                                tunnel: w190 -> [w194]
                                tunnel: [w194] -> w186
                                tunnel: [w193] -> w185
                                tunnel: [w192] -> w184
                                tunnel: [w191] -> w181
                                tunnel: w186 -> [w199]
                                tunnel: w185 -> [w198]
                                tunnel: w184 -> [w196]
                                tunnel: [w197] -> w183
                                tunnel: [w201] -> w188
                                tunnel: w183 -> [w201]
                                tunnel: [w200] -> w182
                                frame #0 {
                                n116 = Tick Count (ms)() -> (millisecond timer value=w191:u32)
                                }
                                frame #1 {
                                n117 = call-poly <vilib>:"DAQmx Write.vi"("task/channels in"=w199, "auto start"=TRUE, "data"=w196, "error in"=w198) -> ("error out"=w197:errorcluster)  [unwired: 9 in, 2 out]
                                }
                                frame #2 {
                                n118 = Tick Count (ms)() -> (millisecond timer value=w200:u32)
                                }
                              }
                              n119 = Subtract(x=w182, y=w181) -> (x-y=→"x-y 2":u32)
                            }
                            frame True {
                            }
                          }
                        }
                        frame True {
                        }
                      }
                      "error AO 2" <- w153
                      n120 = Tick Count (ms)() -> (millisecond timer value=w162:u32)
                      n121 = Subtract(x=w162, y=w163) -> (x-y=→"t ciclo effettivo AO 2":u32)
                      n122 = Compound Arithmetic op=OR(w153, w158, w157) -> (w155:bool)
                    }
                    n123 = flat-sequence {
                      tunnel: w145 -> [_]
                      tunnel: w142 -> [w151]
                      frame #0 {
                        n124 = Send Notification(notification=cluster{"boolean":bool, "variant":variant} {"boolean"=FALSE, "variant"=variant}, notifier=w151) -> ()  [unwired: 1 in, 2 out]
                      }
                    }
                  }
                }
              }
            }
          }
        }
        frame Enabled {
        }
      }
      n125 = disable-structure shown="Enabled" {
        disable-tunnel: w107 -> [w296 _]
        disable-tunnel: w82 -> [w295 _]
        frame Disabled {
          n126 = while {
            tunnel: w295 -> [w302]
            tunnel: w296 -> [w301]
            stop <- w298 stop-if-true
            n127 = Wait on Notification(notifier=w301) -> (notifier out=w297:refnum<notifier>, notification=w300:cluster{"boolean":bool, "variant":variant})  [unwired: 3 in, 2 out]
            n128 = Unbundle By Name(w300) -> ("boolean"=w299:bool)
            n129 = case shown="True" w299 {
              tunnel: w302 -> [_ w308]
              tunnel: [TRUE w306] -> w298
              tunnel: w297 -> [_ w304]
              frame False {
              }
              frame True {
                n130 = flat-sequence {
                  tunnel: w308 -> [w311]
                  tunnel: [w311] -> w307
                  tunnel: [w309] -> w305
                  tunnel: w304 -> [w309]
                  tunnel: w307 -> [_]
                  tunnel: [w316] -> w306
                  tunnel: w305 -> [w313]
                  frame #0 {
                    n131 = Wait (ms)(milliseconds to wait=u32 500) -> ()  [unwired: 1 out]
                  }
                  frame #1 {
                    # "ACQ 4-20mA"
                    n132 = local read "Cluster TASK"() -> (w315:T9)
                    n133 = Unbundle By Name(w315) -> ("AI task 4-20mA"=w314:refnum<k21>)
                    n134 = while {
                      shift-right: [w328] -> w312
                      shift-left: _ -> [w332]
                      shift-right: [w330] -> _
                      shift-left: w314 -> [w331]
                      tunnel: [w323] -> w316
                      i -> [w324]
                      stop <- w329 stop-if-true
                      n135 = local read "SampleRate"() -> (w321:dbl)
                      n136 = Divide(x=w321, y=2.0) -> (x/y=w320:dbl)
                      n137 = call-poly <vilib>:"DAQmx Read.vi"("task/channels in"=w331, "number of samples per channel"=w320, "error in"=w332) -> ("task out"=w330:refnum<k21>, "data"=w326:waveform(dbl)[], "error out"=w328:errorcluster)  [unwired: 10 in]
                      "Not filtered 4-20mA" <- w326
                      n138 = call "Filtri segnali PB.vi"("sampling freq: fs"=w321, "Array"="Impostazioni filtri digitali su canali 4-20mA", "data in"=w326) -> ("filtered"=w325:waveform(dbl)[])  [unwired: 8 in]
                      "Filtered 4-20mA" <- w325
                      n139 = global read "EXIT.vi" "EXIT"() -> (w323:bool)
                      n140 = for {
                        tunnel: [w334] -> w327 mode=indexing
                        tunnel: w325 -> [w333] mode=indexing
                        n141 = call-poly <vilib>:"Mean.vi"("X"=w333) -> ("mean"=w334:dbl)  [unwired: 1 out]
                      }
                      "Array" <- w327
                      n142 = Or(x=w328, y=w323) -> (x .or. y?=w329:bool)
                      "Numeric" <- w324
                    }
                    n143 = flat-sequence {
                      tunnel: w313 -> [w317]
                      tunnel: w312 -> [_]
                      frame #0 {
                        n144 = Send Notification(notification=cluster{"boolean":bool, "variant":variant} {"boolean"=FALSE, "variant"=variant}, notifier=w317) -> ()  [unwired: 1 in, 2 out]
                      }
                    }
                  }
                }
              }
            }
          }
        }
        frame Enabled {
        }
      }
      n145 = while {
        tunnel: w87 -> [w402]
        tunnel: w82 -> [w400]
        stop <- w401 stop-if-true
        n146 = Wait on Notification(notifier=w402) -> (notifier out=w399:refnum<notifier>, notification=w404:cluster{"boolean":bool, "variant":variant})  [unwired: 3 in, 2 out]
        n147 = Unbundle By Name(w404) -> ("boolean"=w403:bool)
        n148 = case shown="True" w403 {
          tunnel: [TRUE w410] -> w401
          tunnel: w400 -> [_ w408]
          tunnel: w399 -> [_ w406]
          frame False {
          }
          frame True {
            n149 = flat-sequence {
              tunnel: [w412] -> w409
              tunnel: w408 -> [w412]
              tunnel: [w411] -> w407
              tunnel: w406 -> [w411]
              tunnel: [w418] -> w410
              tunnel: w409 -> [w417]
              tunnel: w407 -> [w414]
              frame #0 {
                n150 = Wait (ms)(milliseconds to wait=u32 500) -> ()  [unwired: 1 out]
              }
              frame #1 {
                w416 = T9 {"DI task"="", "DO task"="", "AI task 4-20mA"="", "AO task 4-20mA"="", "TC task"="", "COUNTER task"="", "AI task 0-10V"="", "AO task 0-10V"=""} ("Cluster TASK")
                w419 = dbl[] [] ("Array out")
                # "137131 1000RPM"
                # "404040"
                n151 = disable-structure shown="Disabled" {
                  disable-tunnel: w417 -> [w446 _]
                  frame Disabled {
                    w447 = 10123 items=["Finite Samples"=10178, "Continuous Samples"=10123, "Hardware Timed Single Point"=12522] ("sample mode")
                    n152 = call-poly <vilib>:"DAQmx Timing.vi"("sample mode"=w447, "rate"="rate") -> ("task out"=w448:refnum<k21>)  [unwired: 12 in, 1 out]
                    n153 = while {
                      tunnel: w448 -> [w498]
                      tunnel: "rate" -> [w476]
                      tunnel: w446 -> [w475]
                      shift-right: [w455] -> _
                      shift-left: TRUE -> [w456]
                      shift-right: [w452] -> _
                      shift-left: _ -> [w453]
                      shift-right: [w451] -> _
                      shift-left: _ -> [w450]
                      stop <- w495 stop-if-true
                      w472 = 25.0  # %
                      n154 = global read "rpm nominali global.vi" "rpm nominali"() -> (w462:dbl)
                      "Server_RPM_Nom" <- w462
                      n155 = Divide(x=w462, y=60.0) -> (x/y=w468:dbl)
                      "F RPM NOM" <- w468
                      n156 = Subtract(x=w468, y="TOLL F-") -> (x-y=w482:dbl)
                      n157 = Add(x=w468, y="toll F+") -> (x+y=w486:dbl)
                      n158 = In Range and Coerce(upper limit=999999.0, x=w482, lower limit=2.0) -> (coerced(x)=w483:dbl)  [unwired: 1 out]
                      n159 = case shown="False" w475 {
                        tunnel: w498 -> [w509 _]
                        tunnel: "number of samples" -> [w508 w511]
                        tunnel: [w507 w518] -> w489
                        tunnel: [w506 w515] -> w488
                        tunnel: w476 -> [_ w510]
                        frame False {
                          n160 = call-poly <vilib>:"DAQmx Read.vi"("task/channels in"=w509, "number of samples per channel"=w508) -> ("data"=w507:waveform(dbl), "error out"=w506:errorcluster)  [unwired: 11 in, 1 out]
                        }
                        frame True {
                          n161 = Bundle By Name(cluster=cluster{"Fs":dbl, "#s":dbl} {"Fs"=1000.0, "#s"=1000.0} ("sampling info"), "Fs"=w510, "#s"=w511) -> (w516:cluster{"Fs":dbl, "#s":dbl})
                          n162 = call <vilib>:"Uniform White Noise Waveform.vi"("sampling info"=w516, "amplitude"=0.05) -> ("error out"=w515:errorcluster, "signal out"=w519:waveform(dbl))  [unwired: 8 in]
                          n163 = call <vilib>:"Multitone Generator.vi"("sampling info"=w516, "reset signal"=TRUE, "tone amplitudes"="tone amplitudes", "tone frequencies"="tone frequencies") -> ("signal out"=w520:waveform(dbl))  [unwired: 4 in, 3 out]
                          n164 = Add(1:w519, 2:w520) -> (0:w518:waveform(dbl))  [unwired: 1 in, 1 out]
                        }
                      }
                      n165 = Bundle By Name(cluster=cluster{"start":dbl, "stop":dbl} {"start"=15.0, "stop"=40.0} ("frequency range [Hz]"), "start"=w483, "stop"=w486) -> (w485:cluster{"start":dbl, "stop":dbl})
                      "frequency range [Hz]" <- w485
                      n166 = case shown="No Error" w488 {
                        selector: w488 -> [w548 w570]
                        tunnel: "peak search settings" -> [w552 _]
                        tunnel: "channel info" -> [w549 _]
                        tunnel: w485 -> [w546 _]
                        tunnel: w489 -> [w547 _]
                        tunnel: [w537 w570] -> w449
                        tunnel: "averaging parameters" -> [w534 _]
                        tunnel: w456 -> [w536 w567]
                        tunnel: [w533 w568] -> w480
                        tunnel: [w531 w567] -> w455
                        tunnel: [w530 w566] -> w452
                        tunnel: w453 -> [w529 w566]
                        frame No Error {
                          # "5"
                          # "4"
                          # "3"
                          n167 = call-poly <vilib>:"SVL Scale Voltage to EU.vi"("error in (no error)"=w548, "channel info"=w549, "signal [V]"=w547) -> ("scaled signal [EU]"=w550:waveform(dbl))  [unwired: 6 in, 2 out]
                          n168 = call-poly <vilib>:"SVFA Power Spectrum Subset.vi"("scaled signal [EU]"=w550, "window"="window", "frequency range"=w546, "dB On (T)"="dB On (T)", "averaging parameters"=w534, "restart averaging (F)"=w536) -> ("averaging done"=w535:bool, "averages completed"=w527:dbl, "power spectrum [dB EU]"=w542:cluster{"f0":dbl, "df":dbl, "magnitude":dbl[]}, "unit label"=w538:string, "spectrum info"=w544:T24, "error out"=w545:errorcluster)  [unwired: 8 in]
                          "Power Spectrum" <- w542
                          "averaging done" <- w535
                          "averages completed" <- w527
                          n169 = call-poly <vilib>:"SVFA Spectrum Peak Search.vi"("spectrum"=w542, "peak search settings"=w552, "spectrum info in"=w544, "error in (no error)"=w545) -> ("peaks"=w541:cluster{"freq. or order":dbl, "value":dbl}[], "number of peaks"=→"number of peaks":i32, "error out"=w537:errorcluster)  [unwired: 11 in, 2 out]
                          n170 = for "For each peak found" {
                            tunnel: w541 -> [w565] mode=indexing
                            tunnel: [w564] -> w540 mode=indexing
                            tunnel: [w562] -> w539 mode=indexing
                            tunnel: [w560] -> w533 mode=indexing
                            w561 = i16 2 ("precision (6)")
                            # "6"
                            n171 = Unbundle By Name(w565) -> ("freq. or order"=w560:dbl, "value"=w563:dbl)
                            n172 = Number To Fractional String(number=w560, precision (6)=w561) -> (F-format string=w564:string)  [unwired: 2 in]
                            n173 = Number To Fractional String(number=w563, precision (6)=w561) -> (F-format string=w562:string)  [unwired: 2 in]
                          }
                          n174 = property on="Power Spectrum" class="WFGraph (strict)"("Y Scale.Name Label.Text"=w538) -> ()  [unwired: 2 in, 2 out]
                          n175 = Unbundle By Name(w534) -> ("number of averages"=w528:u32)
                          n176 = Greater Or Equal?(x=w527, y=w528) -> (x >= y?=w531:bool)
                          n177 = Equal?(x=w527, y=w528) -> (x = y?=w526:bool)
                          "x = y?" <- w526
                          n178 = case shown="True" w535 {
                            tunnel: w540 -> [_ w559]
                            tunnel: w539 -> [_ w556]
                            frame False {
                            }
                            frame True {
                              n179 = Build Array(w559, w556) -> (w558:string[][])
                              n180 = Transpose 2D Array(2D array=w558) -> (transposed array=w557:string[][])
                              n181 = property on="peaks found" class="MCListbox (strict)"("Item Names"=w557, "Column Header Strings[]"=string[] ["Frequency (Hz)", "Value"] ("Column Header Strings"), "Number of Columns"=u32 2 ("Num Columns")) -> ()  [unwired: 2 in, 2 out]
                            }
                          }
                          n182 = Index Array(array=w533) -> (element=w532:dbl)  [unwired: 1 in]
                          n183 = Select(t=w532, s=w526, f=w529) -> (s? t:f=w530:dbl)
                        }
                        frame Error {
                          n184 = Build Array(-1.0 ("freq. or order")) -> (w568:dbl[])
                        }
                      }
                      n185 = Unbundle By Name("averaging parameters") -> ("averaging mode"=w460:T20)
                      n186 = Not Equal?(x=w460, y=T20."No averaging") -> (x != y?=w458:bool)
                      n187 = Sort 1D Array(array=w480) -> (sorted array=w478:dbl[])
                      n188 = for {
                        tunnel: w462 -> [w524]
                        tunnel: w478 -> [w525] mode=indexing
                        tunnel: [w522] -> w479 mode=indexing
                        n189 = Subtract(x=w525, y=w524) -> (x-y=w523:dbl)
                        n190 = Absolute Value(x=w523) -> (abs(x)=w522:dbl)
                      }
                      n191 = Multiply(x=w462, y=w472) -> (x*y=w471:dbl)
                      n192 = local read "stop"() -> (w495:bool)
                      n193 = Array Max & Min(array=w479) -> (min index (indices)=w477:i32)  [unwired: 3 out]
                      n194 = Index Array(array=w478, index=w477) -> (element=w454:dbl)
                      n195 = Select(t=w452, s=w458, f=w454) -> (s? t:f=w457:dbl)
                      "detected frequency" <- w457
                      n196 = Multiply(x=w457, y=60.0) -> (x*y=w464:dbl)
                      n197 = Subtract(x=w464, y=w462) -> (x-y=w474:dbl)
                      n198 = Absolute Value(x=w474) -> (abs(x)=w473:dbl)
                      n199 = Divide(x=w471, y=100.0) -> (x/y=w469:dbl)
                      n200 = Less Or Equal?(x=w473, y=w469) -> (x <= y?=w465:bool)
                      n201 = case shown="Error" w449 {
                        tunnel: w449 -> [_ w502]
                        tunnel: [FALSE w501] -> w451
                        tunnel: w450 -> [_ w500]
                        frame No Error {
                        }
                        frame Error {
                          n202 = case shown="False" w500 {
                            selector: w500 -> [_ w505]
                            tunnel: w502 -> [w504 _]
                            tunnel: [TRUE w505] -> w501
                            frame False {
                              n203 = call <vilib>:"Simple Error Handler.vi"("error in (no error)"=w504) -> ()  [unwired: 4 in, 5 out]
                            }
                            frame True {
                            }
                          }
                        }
                      }
                      n204 = feedback #1() -> (w466:dbl)  [unwired: 1 in]
                      n205 = Select(t=w464, s=w465, f=w466) -> (s? t:f=w467:dbl)
                      n206 = feedback-in #1(w467) -> ()
                      n207 = Select(t=w464, s=w465, f=w466) -> (s? t:f=→"RPM":dbl)
                    }
                  }
                  frame Enabled {
                  }
                }
                n208 = flat-sequence {
                  tunnel: w416 -> [_]
                  tunnel: w416 -> [w610]
                  tunnel: [w610] -> w420
                  frame #0 {
                    "Stopped" <- FALSE ("Stop")
                  }
                }
                n209 = disable-structure shown="Disabled" {
                  disable-tunnel: w420 -> [w422 _]
                  disable-tunnel: [w421 _] -> w415
                  frame Disabled {
                    n210 = while {
                      tunnel: w422 -> [w431]
                      tunnel: [w423] -> w421
                      stop <- w424 stop-if-true
                      n211 = local read "Cluster TASK"() -> (w429:T9)
                      n212 = Wait (ms)(milliseconds to wait=u32 1000) -> ()  [unwired: 1 out]
                      n213 = Equal?(x=w429, y=w431) -> (x = y?=w425:bool)
                      n214 = case shown="False" w425 {
                        tunnel: w429 -> [w435 _]
                        tunnel: [w434 w437] -> w427
                        tunnel: [w432 _] -> w423
                        frame False {
                          n215 = Unbundle By Name(w435) -> ("TC task"=w433:refnum<k21>)
                          n216 = call-poly <vilib>:"DAQmx Read.vi"("task/channels in"=w433) -> ("data"=w434:dbl[], "error out"=w432:errorcluster)  [unwired: 12 in, 1 out]
                          "error TC" <- w432
                        }
                        frame True {
                          n217 = for {
                            N: 4 -> [_]
                            tunnel: [w439] -> w437 mode=indexing
                            n218 = call "MEASURE SIMULATOR.vi"("delay (100)"=u32 0, "precision %"=0.01, "amplitude"=20.0) -> ("value"=w439:dbl)  [unwired: 8 in]
                          }
                        }
                      }
                      n219 = local read "EXIT 2"() -> (w430:bool)
                      n220 = Array To Cluster(array=w427) -> (cluster=→"Temperature [°C]":T28)
                      n221 = Or(x=w423, y=w430) -> (x .or. y?=w424:bool)
                    }
                  }
                  frame Enabled {
                  }
                }
                n222 = while {
                  tunnel: w416 -> [w592]
                  shift-right: [w591] -> _
                  shift-left: w419 -> [w588]
                  tunnel: w419 -> [w587]
                  shift-right: [w583] -> _
                  shift-left: _ -> [w580]
                  tunnel: [w574] -> w418
                  stop <- w574 stop-if-true
                  # "PENTAIR 30 IMPULSI GIRO"
                  # "PASSO LA FREQUENZA, la conversione viene fatta\nin mappa misure.vi (tors. 60 impulsi giro, sonda 1)"
                  n223 = local read "Cluster TASK"() -> (w577:T9)
                  n224 = Equal?(x=w577, y=w592) -> (x = y?=w573:bool)
                  n225 = case shown="False" w573 {
                    tunnel: w577 -> [w599 _]
                    tunnel: [w597 w605] -> w572
                    tunnel: [w593 _] -> w589
                    frame False {
                      n226 = Unbundle By Name(w599) -> ("COUNTER task"=w596:refnum<k21>)
                      n227 = case shown="True" "Boolean" {
                        tunnel: w596 -> [w600 w604]
                        tunnel: [w600 w603] -> w595
                        frame False {
                        }
                        frame True {
                          n228 = property class="DAQmx Channel"(reference=w604, "CI.Freq.DigFltr.Enable"="DI.DigFltr.Enable", "CI.Freq.DigFltr.MinPulseWidth"="DI.DigFltr.MinPulseWidth") -> (reference out=w603:refnum<k21>)  [unwired: 1 in, 1 out]
                        }
                      }
                      n229 = call-poly <vilib>:"DAQmx Read.vi"("task/channels in"=w595, "timeout"="timeout") -> ("data"=w597:dbl, "error out"=w593:errorcluster)  [unwired: 11 in, 1 out]
                      "CTR error 2" <- w593
                      n230 = call <vilib>:"Clear Errors.vi"("error in (no error)"=w593) -> ()  [unwired: 5 in, 2 out]
                    }
                    frame True {
                      n231 = Random Number (0-1)() -> (number: 0 to 1=w606:dbl)
                      n232 = Add(x=1480.0, y=w606) -> (x+y=w605:dbl)
                      n233 = call "MEASURE SIMULATOR.vi"("precision %"=0.0, "amplitude"=49.5) -> ()  [unwired: 9 in, 1 out]
                    }
                  }
                  "Frequenza" <- w572
                  n234 = Select(t=w587, s=w589, f=w588) -> (s? t:f=w586:dbl[])
                  n235 = local read "EXIT 2"() -> (w574:bool)
                  n236 = In Range and Coerce(upper limit="upper limit", x=w572, lower limit="lower limit") -> (In Range?=w584:bool)  [unwired: 1 out]
                  n237 = Greater?(x=w572, y="upper limit") -> (0:w581:bool)
                  n238 = Select(t=w580, s=w581, f=0.0) -> (s? t:f=w579:dbl)
                  n239 = Select(t=w572, s=w584, f=w579) -> (s? t:f=w583:dbl)
                  n240 = call "media su acquisizioni.vi"("n°campioni"="campioni media rpm", "Array ing"=w586, "Value"=w583) -> ("Array out"=w591:dbl[], "Media"=w571:dbl)  [unwired: 5 in, 2 out]
                  "frequency" <- w571
                  n241 = Build Array(w571, w571) -> (w576:dbl[])
                  n242 = Array To Cluster(array=w576) -> (cluster=→"Contatori [rpm]":cluster{"[0]":dbl, "[1]":dbl})
                }
                n243 = flat-sequence {
                  tunnel: w414 -> [w442]
                  tunnel: w415 -> [_]
                  frame #0 {
                    n244 = Send Notification(notification=cluster{"boolean":bool, "variant":variant} {"boolean"=FALSE, "variant"=variant}, notifier=w442) -> ()  [unwired: 1 in, 2 out]
                  }
                }
              }
            }
          }
        }
      }
      n245 = disable-structure shown="Disabled" {
        frame Disabled {
          (unwired) 20000.0 ("rate")
          n246 = call "NI 9205.vi"() -> ()  [unwired: 18 in, 2 out]
          n247 = call "NI 9263 DOUBLE TASK.vi"() -> ()  [unwired: 10 in, 2 out]
          n248 = call "NI 9265 DOUBLE TASK.vi"() -> ()  [unwired: 10 in, 2 out]
          n249 = call "NI 9215.vi"() -> ()  [unwired: 18 in, 2 out]
        }
        frame Enabled {
        }
      }
      n250 = while {
        shift-right: [w621] -> _
        shift-left: _ -> [w638]
        shift-right: [w636] -> w119
        shift-left: _ -> [w635]
        shift-right: [w633] -> _
        shift-left: "error in (no error)" -> [w634]
        tunnel: w118 -> [w631]
        tunnel: w117 -> [w632]
        tunnel: [w612] -> w120
        shift-right: [w626] -> _
        shift-left: _ -> [w625]
        tunnel: w82 -> [w624]
        shift-right: [w613] -> w80
        shift-left: "error in (no error)" -> [w622]
        tunnel: w110 -> [_]
        tunnel: w107 -> [w620]
        tunnel: w104 -> [w619]
        tunnel: w101 -> [w618]
        tunnel: w102 -> [w617]
        tunnel: w87 -> [w615]
        tunnel: w83 -> [w614]
        stop <- w612 stop-if-true
        # "PROCESSI CONTINUI"
        n251 = Dequeue Element(queue=w631, error in (no error)=w632) -> (queue out=w616:refnum<queue>, element=w630:cluster{"String":string, "variant":variant})  [unwired: 1 in, 2 out]
        n252 = call "loop timer.vi"("millisecond timer IN"=w638) -> ("millisecond timer OUT"=w621:u32, "LOOP TIME (ms)"=→"LOOP TIME (ms)":u32)  [unwired: 9 in]
        n253 = Unbundle(w630) -> ("String"=w629:string, "variant"=w628:variant)
        "STATO" <- w629
        n254 = global read "Globals.vi" "NM?"() -> (w623:bool)
        n255 = case shown="\"INITIALIZE\"" w629 {
          tunnel: [_ _ _ _ _ TRUE] -> w627
          tunnel: [w643 w659 w773 w830 w834 w841] -> w636
          tunnel: w635 -> [w643 _ w773 w830 w834 w841]
          tunnel: w634 -> [w642 w658 w768 w829 w835 w838]
          tunnel: [w642 w645 w739 w829 w835 w838] -> w633
          tunnel: w628 -> [w640 _ _ w827 _ _]
          tunnel: [w641 w651 w766 w828 w833 w840] -> w626
          tunnel: w625 -> [w641 _ w766 w828 w833 w840]
          tunnel: w624 -> [_ w649 w764 _ _ w839]
          tunnel: w623 -> [_ w657 _ _ _ _]
          tunnel: [w639 w653 w765 w807 w831 w836] -> w613
          tunnel: w622 -> [w639 w656 _ w807 w831 w837]
          tunnel: w620 -> [_ w655 _ _ _ _]
          tunnel: w619 -> [_ w654 _ _ _ _]
          tunnel: w618 -> [_ _ _ _ _ _]
          tunnel: w617 -> [_ _ _ _ _ _]
          tunnel: w616 -> [_ w652 w740 _ _ _]
          tunnel: w615 -> [_ w647 _ _ _ _]
          tunnel: w614 -> [_ w648 _ _ _ _]
          frame "NO STATE", Default {
            "variant" <- w640
          }
          frame "INITIALIZE" {
            # "NI READ"
            n256 = case shown="True" TRUE {
              tunnel: [_ w679] -> w651
              tunnel: w658 -> [w661 w666]
              tunnel: [w662 w664] -> w653
              tunnel: w657 -> [_ w678]
              tunnel: w657 -> [_ _]
              tunnel: w656 -> [w662 _]
              tunnel: [w661 w666] -> w645
              tunnel: w655 -> [_ w677]
              tunnel: w654 -> [_ w676]
              tunnel: w649 -> [_ w670]
              tunnel: w652 -> [w660 w663]
              tunnel: w647 -> [_ w675]
              tunnel: w648 -> [_ w668]
              tunnel: [w660 w663] -> w644
              frame False {
              }
              frame True {
                w667 = cluster{"boolean":bool, "variant":variant} {"boolean"=TRUE, "variant"=variant} ("notification")
                n257 = case shown="False" w670 {
                  tunnel: [w699 _] -> w679
                  tunnel: w678 -> [w694 _]
                  tunnel: [w693 _] -> w664
                  tunnel: [w692 _] -> w674
                  frame False {
                    w697 = "/" ("string")
                    n258 = while {
                      tunnel: "C2019010PM" ("RICERCA cDAQ") -> [w711]
                      tunnel: [w710] -> w691
                      shift-right: [FALSE] -> _
                      shift-left: TRUE -> [w704]
                      stop <- w705 stop-if-true
                      n259 = call "Elapsed Time"("Time Target (s)"=45.0, "Reset"=w704, "Auto Reset"=FALSE) -> ("Time has Elapsed"=w706:bool)  [unwired: 9 in, 7 out]
                      n260 = call "FIND_MOD_NAMES.vi"("RICERCA cDAQ"=w711) -> ("error out"=w700:errorcluster, "Array ALIAS"=w709:string[], "Array nomi moduli"=w710:string[])  [unwired: 7 in, 1 out]
                      n261 = Not Equal?(x=w709, y=string[] []) -> (x != y?=w707:bool)
                      n262 = call <vilib>:"Clear Errors.vi"("error in (no error)"=w700) -> ()  [unwired: 5 in, 2 out]
                      n263 = Or(x=w707, y=w706) -> (x .or. y?=w705:bool)
                    }
                    "Array nomi moduli" <- w691
                    n264 = Index Array(array=w691) -> (element #1=w688:string, element #2=w698:string)  [unwired: 8 in, 6 out]
                    n265 = Concatenate Strings(w697, w688, w697, "PFI0" ("string")) -> (w695:string)
                    n266 = flat-sequence {
                      tunnel: [w724] -> w699
                      tunnel: w698 -> [w717]
                      tunnel: w695 -> [w725]
                      tunnel: w694 -> [_]
                      tunnel: [w719] -> w693
                      tunnel: [w719] -> w692
                      tunnel: w688 -> [w722]
                      frame #0 {
                        w715 = 10123 items=["Finite Samples"=10178, "Continuous Samples"=10123, "Hardware Timed Single Point"=12522] ("sample mode")
                        n267 = local read "SampleRate"() -> (w712:dbl)
                        n268 = call "NI 9215.vi"("sample mode"=w715, "MODULE 3 (0-10V)"=w717, "rate"=w712) -> ("task out"=w718:refnum<k21>, "error out"=w716:errorcluster)  [unwired: 15 in]
                        "NI9215" <- w716
                        n269 = disable-structure shown="Enabled" {
                          disable-tunnel: [w734 _] -> _
                          disable-tunnel: w716 -> [w733 _]
                          disable-tunnel: w715 -> [w732 _]
                          disable-tunnel: [w731 _] -> w713
                          disable-tunnel: w712 -> [w730 _]
                          frame Disabled {
                            n270 = call "NI 9203 DOUBLE TASK.vi"("sample mode"=w732, "rate"=w730, "error in"=w733) -> ("task out"=w734:refnum<k21>, "error out"=w731:errorcluster)  [unwired: 15 in]
                          }
                          frame Enabled {
                          }
                        }
                        "NI9203" <- w713
                        n271 = disable-structure shown="Enabled" {
                          disable-tunnel: [w729 _] -> _
                          disable-tunnel: [w728 _] -> w714
                          disable-tunnel: w713 -> [w727 _]
                          frame Disabled {
                            n272 = call "NI 9211_TASK_TC.vi"("error in"=w727) -> ("error out"=w728:errorcluster, "task out"=w729:refnum<k21>)  [unwired: 9 in]
                          }
                          frame Enabled {
                          }
                        }
                        "NI9265" <- w714
                        n273 = call "NI 9411 TASK.vi"("divisor"=u32 4, "error in"=w714, "CI.Freq.Term"=w725, "MODULE NAME"=w722) -> ("error out"=w720:errorcluster, "task out"=w721:refnum<k21>)  [unwired: 6 in]
                        "CTR TASK" <- w720
                        n274 = Merge Errors(w716, w713, w714, w720) -> (w719:errorcluster)
                        n275 = Bundle By Name(cluster=T9 {"DI task"="", "DO task"="", "AI task 4-20mA"="", "AO task 4-20mA"="", "TC task"="", "COUNTER task"="", "AI task 0-10V"="", "AO task 0-10V"=""} ("Cluster TASK"), "AI task 0-10V"=w718, "COUNTER task"=w721) -> (w724:T9)
                        n276 = call <vilib>:"Clear Errors.vi"("error in (no error)"=w719) -> ()  [unwired: 5 in, 2 out]
                      }
                    }
                  }
                  frame True {
                  }
                }
                n277 = call <vilib>:"Clear Errors.vi"("error in (no error)"=w674) -> ("error out"=w672:errorcluster)  [unwired: 5 in, 1 out]
                n278 = Send Notification(notification=w667, notifier=w677, error in (no error)=w672) -> (error out=w673:errorcluster)  [unwired: 1 out]
                n279 = disable-structure shown="Enabled" {
                  disable-tunnel: w676 -> [w686 _]
                  disable-tunnel: w673 -> [w685 w687]
                  disable-tunnel: [w684 w687] -> w671
                  disable-tunnel: w667 -> [w683 _]
                  frame Disabled {
                    n280 = Send Notification(notification=w683, notifier=w686, error in (no error)=w685) -> (error out=w684:errorcluster)  [unwired: 1 out]
                  }
                  frame Enabled {
                  }
                }
                n281 = Send Notification(notification=w667, notifier=w675, error in (no error)=w671) -> (error out=w669:errorcluster)  [unwired: 1 out]
                n282 = disable-structure shown="Disabled" {
                  disable-tunnel: w669 -> [w682 _]
                  disable-tunnel: w668 -> [w681 _]
                  disable-tunnel: w667 -> [w680 _]
                  frame Disabled {
                    n283 = Send Notification(notification=w680, notifier=w681, error in (no error)=w682) -> ()  [unwired: 2 out]
                  }
                  frame Enabled {
                  }
                }
                n284 = call "SEND STATUS.vi"("ELEMENT"=DEVICE_NAME."NI cDAQ", "error in (no error)"=w664) -> ()  [unwired: 9 in, 1 out]
              }
            }
            "error in (no error) 2" <- w653
            "Cluster TASK" <- w651
            n285 = control-ref of="This VI"() -> (w659:refnum<vi>)
            n286 = Enqueue Element(queue=w644, element=cluster{"String":string, "variant":variant} {"String"="NI READ", "variant"=variant}) -> ()  [unwired: 2 in, 3 out]
          }
          frame "NI READ" {
            w763 = T7 {"AI (0-10V)"={"AI 0"=0.0, "AI 1"=0.0, "AI 2"=0.0, "AI 3"=0.0, "AI 4"=0.0, "AI 5"=0.0, "AI 6"=0.0, "AI 7"=0.0, "AI 8"=0.0, "AI 9"=0.0, "AI 10"=0.0, "AI 11"=0.0, "AI 12"=0.0, "AI 13"=0.0, "AI 14"=0.0, "AI 15"=0.0, "AI 16"=0.0, "AI 17"=0.0, "AI 18"=0.0, "AI 19"=0.0, "AI 20"=0.0, "AI 21"=0.0, "AI 22"=0.0, "AI 23"=0.0, "AI 24"=0.0, "AI 25"=0.0, "AI 26"=0.0, "AI 27"=0.0, "AI 28"=0.0, "AI 29"=0.0, "AI 30"=0.0, "AI 31"=0.0}, "StatoAO_Cdaq[0-10V]"={"AO 1"=0.0, "AO 2"=0.0, "AO 3"=0.0, "AO 4"=0.0}, "Contatori [rpm]"={"RPM 1"=0.0, "RPM 2"=0.0}, "StatoAO_Cdaq [4-20mA]"={"Cdaq_AO [0-10V] 0"=0.0, "Cdaq_AO [0-10V] 1"=0.0, "Cdaq_AO [0-10V] 2"=0.0, "Cdaq_AO [0-10V] 3"=0.0, "Cdaq_AO [4-20mA] 0"=0.0, "Cdaq_AO [4-20mA] 1"=0.0, "Cdaq_AO [4-20mA] 2"=0.0, "Cdaq_AO [4-20mA] 3"=0.0, "Cdaq_AO [4-20mA] 4"=0.0, "Cdaq_AO [4-20mA] 5"=0.0, "Cdaq_AO [4-20mA] 6"=0.0, "Cdaq_AO [4-20mA] 7"=0.0}, "StatoDO_Cdaq"={"Scorta 0"=FALSE, "Scorta 1"=FALSE, "Scorta 2"=FALSE, "Scorta 3"=FALSE, "Scorta 4"=FALSE, "Scorta 5"=FALSE, "Scorta 6"=FALSE, "Scorta 7"=FALSE, "Scorta 8"=FALSE, "Scorta 9"=FALSE, "Scorta 10"=FALSE, "Scorta 11"=FALSE, "Scorta 12"=FALSE, "Scorta 13"=FALSE, "Scorta 14"=FALSE, "Scorta 15"=FALSE, "Scorta 16"=FALSE, "Scorta 17"=FALSE, "Scorta 18"=FALSE, "Scorta 19"=FALSE, "Scorta 20"=FALSE, "Scorta 21"=FALSE, "Scorta 22"=FALSE, "Scorta 23"=FALSE, "Scorta 24"=FALSE, "Scorta 25"=FALSE, "Scorta 26"=FALSE, "Scorta 27"=FALSE, "Scorta 28"=FALSE, "Scorta 29"=FALSE, "Scorta 30"=FALSE, "Scorta 31"=FALSE}, "DI"={"Scorta 0"=FALSE, "Scorta 1"=FALSE, "Scorta 2"=FALSE, "Scorta 3"=FALSE, "Scorta 4"=FALSE, "Scorta 5"=FALSE, "Scorta 6"=FALSE, "Scorta 7"=FALSE, "Scorta 8"=FALSE, "Scorta 9"=FALSE, "Scorta 10"=FALSE, "Scorta 11"=FALSE, "Scorta 12"=FALSE, "Scorta 13"=FALSE, "Scorta 14"=FALSE, "Scorta 15"=FALSE, "Scorta 16"=FALSE, "Scorta 17"=FALSE, "Scorta 18"=FALSE, "Scorta 19"=FALSE, "Scorta 20"=FALSE, "Scorta 21"=FALSE, "Scorta 22"=FALSE, "Scorta 23"=FALSE, "Scorta 24"=FALSE, "Scorta 25"=FALSE, "Scorta 26"=FALSE, "Scorta 27"=FALSE, "Scorta 28"=FALSE, "Scorta 29"=FALSE, "Scorta 30"=FALSE, "Scorta 31"=FALSE}, "AI (4-20mA)"={"AI 0"=0.0, "AI 1"=0.0, "AI 2"=0.0, "AI 3"=0.0, "AI 4"=0.0, "AI 5"=0.0, "AI 6"=0.0, "AI 7"=0.0, "AI 8"=0.0, "AI 9"=0.0, "AI 10"=0.0, "AI 11"=0.0, "AI 12"=0.0, "AI 13"=0.0, "AI 14"=0.0, "AI 15"=0.0}, "TC [°C]"={"tc 1"=0.0, "tc 2"=0.0, "tc 3"=0.0, "tc 4"=0.0}}  # Cluster READ
            n287 = case shown="False" w764 {
              tunnel: w766 -> [w786 _]
              tunnel: [w785 _] -> w742
              tunnel: [w780 w790] -> w761
              tunnel: [w776 _] -> _
              frame False {
                n288 = Unbundle By Name(w786) -> ("AI task 0-10V"=w783:refnum<k21>)
                n289 = local read "N°samples"() -> (w782:i32)
                n290 = local read "SampleRate"() -> (w784:dbl)
                n291 = call-poly <vilib>:"DAQmx Read.vi"("task/channels in"=w783, "number of samples per channel"=w782) -> ("data"=w776:waveform(dbl)[], "error out"=w785:errorcluster)  [unwired: 11 in, 1 out]
                "Not filtered 0-10V" <- w776
                "error out 3" <- w785
                n292 = call "Filtri segnali PB.vi"("sampling freq: fs"=w784, "Array"="Impostazioni filtri digitali su canali 0-10V", "data in"=w776) -> ("filtered"=w778:waveform(dbl)[])  [unwired: 8 in]
                "Filtered 0-10V" <- w778
                n293 = for {
                  tunnel: [w788] -> w781 mode=indexing
                  tunnel: w778 -> [w787] mode=indexing
                  n294 = call-poly <vilib>:"Mean.vi"("X"=w787) -> ("mean"=w788:dbl)  [unwired: 1 out]
                }
                n295 = local read "Array"() -> (w779:dbl[])
                n296 = Build Array (concatenate)(w781, w779) -> (w780:dbl[])
              }
              frame True {
                n297 = for {
                  N: 16 -> [_]
                  tunnel: [w803] -> w794 mode=indexing
                  n298 = Random Number (0-1)() -> (number: 0 to 1=w806:dbl)
                  n299 = Divide(x=w806, y=50.0) -> (x/y=w805:dbl)
                  n300 = In Range and Coerce(upper limit=0.02, x=w805, lower limit=0.004) -> (coerced(x)=w803:dbl)  [unwired: 1 out]
                }
                n301 = for {
                  N: 4 -> [_]
                  tunnel: [w797] -> w789 mode=indexing
                  n302 = Random Number (0-1)() -> (number: 0 to 1=w800:dbl)
                  n303 = Divide(x=w800, y=0.1) -> (x/y=w799:dbl)
                  n304 = In Range and Coerce(upper limit=10.0, x=w799, lower limit=-10.0) -> (coerced(x)=w797:dbl)  [unwired: 1 out]
                }
                n305 = Wait (ms)(milliseconds to wait=u32 500) -> ()  [unwired: 1 out]
                n306 = Build Array (concatenate)(w794, w789) -> (w790:dbl[])
              }
            }
            n307 = Merge Errors(w742) -> (w765:errorcluster)
            n308 = local read "Contatori [rpm]"() -> (w746:cluster{"RPM 1":dbl, "RPM 2":dbl})
            n309 = local read "AO cdaq 4-20mA"() -> (w762:T1)
            n310 = local read "AO cdaq [0-10V]"() -> (w751:T1)
            n311 = feedback-in #2(w742) -> ()
            n312 = feedback #2() -> (w743:errorcluster)  [unwired: 1 in]
            n313 = local read "Temperature [°C]"() -> (w735:T5)
            n314 = Not Equal?(x=w743, y=w742) -> (x != y?=w741:bool)
            n315 = local read "Array"() -> (w745:dbl[])
            n316 = case shown="True" w741 {
              tunnel: w742 -> [_ w774]
              frame False {
              }
              frame True {
                n317 = call "SEND STATUS.vi"("ELEMENT"=DEVICE_NAME."NI cDAQ", "error in (no error)"=w774) -> ()  [unwired: 9 in, 1 out]
              }
            }
            n318 = Array To Cluster(array=w745) -> (cluster=w744:T29)
            n319 = Array To Cluster(array=w761) -> (cluster=w760:T30)
            n320 = Unbundle By Name(w751) -> ("[0]"=w750:dbl, "[1]"=w749:dbl, "[2]"=w748:dbl, "[3]"=w747:dbl)
            n321 = Unbundle By Name(w762) -> ("[0]"=w759:dbl, "[1]"=w758:dbl, "[2]"=w757:dbl, "[3]"=w756:dbl, "[4]"=w755:dbl, "[5]"=w754:dbl, "[6]"=w753:dbl, "[7]"=w752:dbl)
            n322 = Bundle By Name(cluster=w763, "AI (4-20mA)"=w744, "AI (0-10V)"=w760, "Contatori [rpm]"=w746, "TC [°C]"=w735, "StatoAO_Cdaq [4-20mA].Cdaq_AO [0-10V] 0"=w750, "StatoAO_Cdaq [4-20mA].Cdaq_AO [0-10V] 1"=w749, "StatoAO_Cdaq [4-20mA].Cdaq_AO [0-10V] 2"=w748, "StatoAO_Cdaq [4-20mA].Cdaq_AO [0-10V] 3"=w747, "StatoAO_Cdaq [4-20mA].Cdaq_AO [4-20mA] 0"=w759, "StatoAO_Cdaq [4-20mA].Cdaq_AO [4-20mA] 1"=w758, "StatoAO_Cdaq [4-20mA].Cdaq_AO [4-20mA] 2"=w757, "StatoAO_Cdaq [4-20mA].Cdaq_AO [4-20mA] 3"=w756, "StatoAO_Cdaq [4-20mA].Cdaq_AO [4-20mA] 4"=w755, "StatoAO_Cdaq [4-20mA].Cdaq_AO [4-20mA] 5"=w754, "StatoAO_Cdaq [4-20mA].Cdaq_AO [4-20mA] 6"=w753, "StatoAO_Cdaq [4-20mA].Cdaq_AO [4-20mA] 7"=w752) -> (w767:T7)
            "Cluster READ" <- w767
            n323 = Bundle By Name(cluster=T21 {"Array of elements"=[], "Single element"={"String"="READ NI", "variant"=variant}, "enque at\nopposite end (F)"=FALSE, "no replications (F)"=FALSE} ("Enqueue cluster"), "Single element.variant"=w767) -> (w769:T21)
            n324 = global write "Globals.vi" "NI READ"(w767) -> ()
            n325 = call "SMQ_MANAGER.vi"("Function"=enum16{"INITIALIZE", "ENQUEUE", "STOP ALL"}."ENQUEUE", "Queue name"="DATA_Q", "error in (no error)"=w768, "Enqueue cluster"=w769) -> ("error out"=w739:errorcluster)  [unwired: 7 in]
            n326 = Select(t=cluster{"String":string, "variant":variant} {"String"="INITIALIZE", "variant"=variant} ("element"), s=w765, f=cluster{"String":string, "variant":variant} {"String"="NI READ", "variant"=variant} ("element")) -> (s? t:f=w736:cluster{"String":string, "variant":variant})
            n327 = Enqueue Element(queue=w740, element=w736) -> ()  [unwired: 2 in, 3 out]
          }
          frame "IMPOSTA AI SIM" {
            w817 = cluster{"Amplitude":dbl, "Precision %":dbl} {"Amplitude"=4.0, "Precision %"=0.01} ("Cluster SIM AI")
            n328 = Variant To Data(type=T22 {"Portata 1"={"Amplitude [mA]"=4.0, "Precision %"=0.01}, "Portata 2"={"Amplitude [mA]"=4.0, "Precision %"=0.01}, "Portata 3"={"Amplitude [mA]"=4.0, "Precision %"=0.01}, "Portata 4"={"Amplitude [mA]"=4.0, "Precision %"=0.01}, "Pressione 1"={"Amplitude [mA]"=4.0, "Precision %"=0.01}, "Pressione 2"={"Amplitude [mA]"=4.0, "Precision %"=0.01}, "Pressione 3"={"Amplitude [mA]"=4.0, "Precision %"=0.01}, "Pressione 4"={"Amplitude [mA]"=4.0, "Precision %"=0.01}, "Velocità"={"Amplitude [mA]"=4.0, "Precision %"=0.01}, "Coppia"={"Amplitude [mA]"=4.0, "Precision %"=0.01}, "Temperatura 1"={"Amplitude [mA]"=4.0, "Precision %"=0.01}, "Temperatura 2"={"Amplitude [mA]"=4.0, "Precision %"=0.01}, "Livello"={"Amplitude [mA]"=4.0, "Precision %"=0.01}, "Pressione serbatoio"={"Amplitude [mA]"=4.0, "Precision %"=0.01}} ("Cluster AI SIM"), Variant=w827) -> (data=w824:T22)  [unwired: 1 in, 1 out]
            n329 = Unbundle By Name(w824) -> ("Portata 1"=w823:cluster{"Amplitude [mA]":dbl, "Precision %":dbl}, "Portata 2"=w822:cluster{"Amplitude [mA]":dbl, "Precision %":dbl}, "Portata 3"=w821:cluster{"Amplitude [mA]":dbl, "Precision %":dbl}, "Portata 4"=w820:cluster{"Amplitude [mA]":dbl, "Precision %":dbl}, "Pressione 1"=w816:cluster{"Amplitude [mA]":dbl, "Precision %":dbl}, "Pressione 2"=w815:cluster{"Amplitude [mA]":dbl, "Precision %":dbl}, "Pressione 3"=w814:cluster{"Amplitude [mA]":dbl, "Precision %":dbl}, "Pressione 4"=w813:cluster{"Amplitude [mA]":dbl, "Precision %":dbl}, "Velocità"=w819:cluster{"Amplitude [mA]":dbl, "Precision %":dbl}, "Coppia"=w818:cluster{"Amplitude [mA]":dbl, "Precision %":dbl}, "Temperatura 1"=w812:cluster{"Amplitude [mA]":dbl, "Precision %":dbl}, "Temperatura 2"=w811:cluster{"Amplitude [mA]":dbl, "Precision %":dbl}, "Livello"=w810:cluster{"Amplitude [mA]":dbl, "Precision %":dbl}, "Pressione serbatoio"=w809:cluster{"Amplitude [mA]":dbl, "Precision %":dbl})
            n330 = Build Array(w823, w822, w821, w820, w819, w818, w817, w817, w816, w815, w814, w813, w812, w811, w810, w809) -> (w808:T31)
            n331 = Replace Array Subset(array=cluster{"Amplitude":dbl, "Precision %":dbl}[] [{"Amplitude"=4.0, "Precision %"=0.01}, {"Amplitude"=4.0, "Precision %"=0.01}, {"Amplitude"=4.0, "Precision %"=0.01}, {"Amplitude"=4.0, "Precision %"=0.01}, {"Amplitude"=4.0, "Precision %"=0.01}, {"Amplitude"=4.0, "Precision %"=0.01}, {"Amplitude"=4.0, "Precision %"=0.01}, {"Amplitude"=4.0, "Precision %"=0.01}, {"Amplitude"=4.0, "Precision %"=0.01}, {"Amplitude"=4.0, "Precision %"=0.01}, {"Amplitude"=4.0, "Precision %"=0.01}, {"Amplitude"=4.0, "Precision %"=0.01}, {"Amplitude"=4.0, "Precision %"=0.01}, {"Amplitude"=4.0, "Precision %"=0.01}, {"Amplitude"=4.0, "Precision %"=0.01}, {"Amplitude"=4.0, "Precision %"=0.01}, {"Amplitude"=4.0, "Precision %"=0.01}, {"Amplitude"=4.0, "Precision %"=0.01}, {"Amplitude"=4.0, "Precision %"=0.01}, {"Amplitude"=4.0, "Precision %"=0.01}, {"Amplitude"=4.0, "Precision %"=0.01}, {"Amplitude"=4.0, "Precision %"=0.01}, {"Amplitude"=4.0, "Precision %"=0.01}, {"Amplitude"=4.0, "Precision %"=0.01}, {"Amplitude"=4.0, "Precision %"=0.01}, {"Amplitude"=4.0, "Precision %"=0.01}, {"Amplitude"=4.0, "Precision %"=0.01}, {"Amplitude"=4.0, "Precision %"=0.01}, {"Amplitude"=4.0, "Precision %"=0.01}, {"Amplitude"=4.0, "Precision %"=0.01}, {"Amplitude"=4.0, "Precision %"=0.01}, {"Amplitude"=4.0, "Precision %"=0.01}, {"Amplitude"=4.0, "Precision %"=0.01}] ("ARRAY SIM AI"), new element=w808) -> ()  [unwired: 1 in, 1 out]
          }
          frame "OPEN" {
            n332 = global read "Globals.vi" "MONITOR 1"() -> (w832:u8)
            n333 = call "easy open VI panel.vi"("Monitor(1)"=w832, "VI in"=w834) -> ()  [unwired: 9 in, 1 out]
          }
          frame "STOP" {
            n334 = case shown="False" w839 {
              tunnel: w840 -> [w855 _]
              tunnel: w837 -> [w845 w856]
              tunnel: [w843 w856] -> w836
              frame False {
                w852 = TRUE  # auto start
                n335 = Unbundle By Name(w855) -> ("AO task 4-20mA"=w853:refnum<k21>, "DO task"=w854:refnum<k21>)
                n336 = Initialize Array(FALSE ("Boolean"), 32 ("dimension size")) -> (w849:bool[])
                n337 = call-poly <vilib>:"DAQmx Write.vi"("task/channels in"=w854, "auto start"=w852, "data"=w849, "error in"=w845) -> ("error out"=w844:errorcluster)  [unwired: 9 in, 2 out]
                n338 = Initialize Array(0.004 ("Waveform"), 16 ("dimension size")) -> (w846:dbl[])
                n339 = call-poly <vilib>:"DAQmx Write.vi"("task/channels in"=w853, "auto start"=w852, "data"=w846, "error in"=w844) -> ("error out"=w843:errorcluster)  [unwired: 9 in, 2 out]
              }
              frame True {
              }
            }
          }
        }
        n340 = Or(x=w613, y=w627) -> (x .or. y?=w612:bool)
      }
      n341 = while {
        stop <- w857 stop-if-true
        # "PROCESSI A EVENTI"
        n342 = event shown="[3] \"SET AO\": Value Change" {
          selector: _ -> [_ _ _ _]
          dyn-events: _ -> [_ _ _ _]
          timeout: _ -> [_ _ _ _]
          tunnel: [w858 _ _ _] -> w857
          event "Stopped": Value Change {
            n343 = event-data() -> ("NewVal"=w858:bool)  [unwired: 1 in]
            n344 = flat-sequence {
              frame #0 {
                n345 = local write "EXIT 2"(TRUE) -> ()
              }
              frame #1 {
                n346 = Wait (ms)(milliseconds to wait=u32 1000) -> ()  [unwired: 1 out]
              }
              frame #2 {
                w865 = dbl[] [0.0]
                w864 = dbl[] [0.0]
                n347 = Obtain Queue(name (unnamed)="SET AO 0-10V CDAQ", element data type=w865) -> (queue out=w866:refnum<queue>, error out=w867:errorcluster)  [unwired: 3 in, 1 out]
                n348 = Obtain Queue(name (unnamed)="SET AO 4-20mA CDAQ", element data type=w864) -> (queue out=w863:refnum<queue>, error out=w862:errorcluster)  [unwired: 3 in, 1 out]
                n349 = Enqueue Element(queue=w866, element=w865, error in (no error)=w867) -> ()  [unwired: 1 in, 3 out]
                n350 = Enqueue Element(queue=w863, element=w864, error in (no error)=w862) -> ()  [unwired: 1 in, 3 out]
              }
            }
          }
          event "SALVA IMP FILTRI 4-20mA": Value Change {
            n351 = event-data() -> ()  [unwired: 1 in, 6 out]
            n352 = local read "Impostazioni filtri digitali su canali 4-20mA"() -> (w873:T10)
            n353 = for {
              tunnel: w873 -> [w884] mode=indexing
              tunnel: [w874] -> w872 mode=indexing
              w878 = i16 2 ("precision (6)")
              n354 = Unbundle By Name(w884) -> ("filter?"=w883:bool, "low cutoff freq: fl"=w880:dbl, "order"=w879:i32)
              n355 = Number To Fractional String(number=w880, precision (6)=w878) -> (F-format string=w876:string)  [unwired: 2 in]
              n356 = Number To Fractional String(number=w879, precision (6)=w878) -> (F-format string=w875:string)  [unwired: 2 in]
              n357 = Select(t="1", s=w883, f="0") -> (s? t:f=w877:string)
              n358 = Build Array(w877, w876, w875) -> (w874:string[])
            }
            n359 = call <vilib>:"Application Directory.vi"() -> ("Application Directory"=w870:path)
            n360 = Build Path(base path=w870, name or relative path="Settings\\Filtri digitali 4-20mA.txt") -> (appended path=w869:path)
            n361 = call-poly <vilib>:"Write To Spreadsheet File.vi"("2D data"=w872, "file path (dialog if empty)"=w869) -> ()  [unwired: 6 in, 1 out]
          }
          event "SALVA IMP FILTRI 0-10V": Value Change {
            n362 = event-data() -> ()  [unwired: 1 in, 6 out]
            n363 = local read "Impostazioni filtri digitali su canali 0-10V"() -> (w889:T10)
            n364 = for {
              tunnel: w889 -> [w900] mode=indexing
              tunnel: [w890] -> w888 mode=indexing
              w894 = i16 2 ("precision (6)")
              n365 = Unbundle By Name(w900) -> ("filter?"=w899:bool, "low cutoff freq: fl"=w896:dbl, "order"=w895:i32)
              n366 = Number To Fractional String(number=w896, precision (6)=w894) -> (F-format string=w892:string)  [unwired: 2 in]
              n367 = Number To Fractional String(number=w895, precision (6)=w894) -> (F-format string=w891:string)  [unwired: 2 in]
              n368 = Select(t="1", s=w899, f="0") -> (s? t:f=w893:string)
              n369 = Build Array(w893, w892, w891) -> (w890:string[])
            }
            n370 = call <vilib>:"Application Directory.vi"() -> ("Application Directory"=w886:path)
            n371 = Build Path(base path=w886, name or relative path="Settings\\Filtri digitali 0-10V.txt") -> (appended path=w885:path)
            n372 = call-poly <vilib>:"Write To Spreadsheet File.vi"("2D data"=w888, "file path (dialog if empty)"=w885) -> ()  [unwired: 6 in, 1 out]
          }
          event "SET AO": Value Change {
            n373 = event-data() -> ()  [unwired: 1 in, 6 out]
            n374 = Obtain Queue(name (unnamed)="SET AO 0-10V CDAQ", element data type=dbl[] []) -> (queue out=w903:refnum<queue>, error out=w902:errorcluster)  [unwired: 3 in, 1 out]
            n375 = Enqueue Element(queue=w903, element="element", error in (no error)=w902) -> ()  [unwired: 1 in, 3 out]
          }
        }
      }
      n376 = disable-structure shown="Disabled" {
        disable-tunnel: w101 -> [w395 _]
        frame Disabled {
          n377 = case shown="True" w395 {
            frame False {
            }
            frame True {
              n378 = while {
                stop <- w398 stop-if-true
                n379 = call "wait for new data from server.vi"() -> ("Letture"=→"Letture":T3)  [unwired: 11 in]
                n380 = global read "EXIT.vi" "EXIT"() -> (w398:bool)
                n381 = Wait (ms)(milliseconds to wait=u32 100) -> ()  [unwired: 1 out]
              }
            }
          }
        }
        frame Enabled {
        }
      }
      n382 = disable-structure shown="Disabled" {
        frame Disabled {
          n383 = while {
            tunnel: _ -> [w346]
            tunnel: _ -> [w345]
            stop <- w342 stop-if-true
            n384 = Wait on Notification(notifier=w345) -> (notification=w344:cluster{"boolean":bool, "variant":variant})  [unwired: 3 in, 3 out]
            n385 = Unbundle By Name(w344) -> ("boolean"=w343:bool)
            n386 = case shown="True" w343 {
              tunnel: w346 -> [_ w349]
              tunnel: [_ w347] -> w342
              frame False {
              }
              frame True {
                n387 = flat-sequence {
                  tunnel: w349 -> [w351]
                  tunnel: [w351] -> w348
                  tunnel: w348 -> [w354]
                  tunnel: [w353] -> w347
                  frame #0 {
                    n388 = Wait (ms)(milliseconds to wait=u32 500) -> ()  [unwired: 1 out]
                  }
                  frame #1 {
                    # "Scrittura 32 DO"
                    n389 = Obtain Queue(name (unnamed)="SET DO CDAQ", element data type=bool[] []) -> (queue out=w358:refnum<queue>, error out=w357:errorcluster)  [unwired: 3 in, 1 out]
                    n390 = while {
                      shift-right: [w377] -> w355
                      shift-left: errorcluster {"status"=FALSE, "code"=0, "source"=""} ("error out") -> [w387]
                      tunnel: w358 -> [w385]
                      tunnel: w357 -> [w386]
                      tunnel: w354 -> [w380]
                      shift-right: [w378] -> _
                      shift-left: bool[] [] -> [w366]
                      tunnel: [w362] -> w353
                      i -> [w383]
                      stop <- w376 stop-if-true
                      w371 = 20  # resistomat ramo 2
                      w372 = 19  # resistomat ramo1
                      w373 = 12  # potenza
                      n391 = Dequeue Element(queue=w385, error in (no error)=w386) -> (queue out=w384:refnum<queue>, element=w363:bool[])  [unwired: 1 in, 2 out]
                      n392 = call <vilib>:"Clear Errors.vi"("error in (no error)"=w387) -> ("error out"=w361:errorcluster)  [unwired: 5 in, 1 out]
                      n393 = Equal?(x=w366, y=w363) -> (x = y?=w364:bool)
                      n394 = Get Queue Status(queue=w384) -> (# elements in queue=→"# pending insert 3":i32)  [unwired: 2 in, 7 out]
                      n395 = local read "Cluster TASK"() -> (w375:T9)
                      n396 = Index Array(array=w363, index #1=w373, index #2=w372, index #3=w371) -> (element #1=w367:bool, element #2=w369:bool, element #3=w370:bool)
                      n397 = Or(x=w369, y=w370) -> (x .or. y?=w368:bool)
                      n398 = Unbundle By Name(w375) -> ("AI task 0-10V"=w374:refnum<k21>)
                      n399 = And(x=w367, y=w368) -> (x .and. y?=w365:bool)
                      n400 = global write "Global allarme combinazione DO.vi" "Allarme combinazione DO"(w365) -> ()
                      n401 = Select(t=w366, s=w365, f=w363) -> ()  [unwired: 1 out]
                      n402 = Array To Cluster(array=w363) -> (cluster=→"statoDO 2":T32)
                      n403 = global read "EXIT.vi" "EXIT"() -> (w362:bool)
                      n404 = Compound Arithmetic op=OR(w364, w380, w362) -> (w379:bool)
                      n405 = case shown="False" w379 {
                        tunnel: w374 -> [w392 _]
                        tunnel: w361 -> [w391 w393]
                        tunnel: [w390 w393] -> w377
                        tunnel: w363 -> [w389 w394]
                        tunnel: [w389 w394] -> w378
                        frame False {
                          n406 = call-poly <vilib>:"DAQmx Write.vi"("task/channels in"=w392, "auto start"=TRUE, "data"=w389, "error in"=w391) -> ("error out"=w390:errorcluster)  [unwired: 9 in, 2 out]
                        }
                        frame True {
                        }
                      }
                      "error DO 2" <- w377
                      n407 = Or(x=w362, y=w362) -> (x .or. y?=w376:bool)
                      "Numeric 2" <- w383
                    }
                    n408 = call <vilib>:"Simple Error Handler.vi"("error in (no error)"=w355) -> ()  [unwired: 4 in, 5 out]
                  }
                }
              }
            }
          }
        }
        frame Enabled {
        }
      }
      n409 = flat-sequence {
        tunnel: w119 -> [w340]
        tunnel: w80 -> [w335]
        frame #0 {
          n410 = property class="VI"(reference=w340) -> (reference out=w336:refnum<vi>, "FP.State"=w339:T19)  [unwired: 1 in, 1 out]
          n411 = Not Equal?(x=T19."Closed", y=w339) -> (x != y?=w337:bool)
          n412 = case shown="True" w337 {
            tunnel: w336 -> [_ w341]
            frame False {
            }
            frame True {
              n413 = invoke class="VI" method="FP.Close"(reference=w341) -> ()  [unwired: 2 in, 3 out]
            }
          }
          "error out" <- w335
        }
      }
      n414 = property on="Stopped" class="Bool (strict)"("Val(Sgnl)"=w120) -> ()  [unwired: 2 in, 2 out]
      "EXIT 2" <- FALSE ("EXIT 2")
    }
  }
